vi "校准UI.vi"() -> ()   [LabVIEW 2016, in "斯坦道多参数.lvlib"]
uses:
  <vilib>/Utility/miscctls.llb/LVPointTypeDef.ctl
  <vilib>/Utility/miscctls.llb/LVPositionTypeDef.ctl
  <vilib>/ptbypt/NI_PtbyPt.lvlib
panel:
  out "溶解氧浓度值":dbl=25.0 caption="检测值：" format="%#.2f mg/L"
  out "电极状态标志":u16
  in  "恢复出厂":bool
  in  "电极系数面板":enum32{"选项卡 1"}(tab)
  out "B":dbl=25.0 caption="电极零点：" format="%#.6f"
  out "K":dbl=25.0 caption="电极系数：" format="%#.6f"
  in  "测试参数面板":enum32{"选项卡 1"}(tab)
  in  "自动盐度补偿":bool caption="自动盐度补偿："
  in  "偏移修正值":dbl=25.0 caption="偏移修正值：" format="%#_6f"
  in  "滤波次数":dbl=25.0 caption="滤波次数：" min=1.0 step=1.0
  in  "测量量程":u16(ring)=1 caption="测量量程："
  in  "盐度":dbl=25.0 caption="盐度：" format="%#_6f"
  in  "大气压力":dbl=25.0 caption="大气压力：" format="%#_6f"
  in  "温度系数":dbl=25.0 caption="温度系数：" format="%#.6f"
  out "信号值":dbl=25.0 caption="信号值：" format="%#.2f mV"
  out "检测值":dbl=25.0 caption="检测值：" format="%#.2f"
  out "序列号":string caption="序列号："
  in  "选项卡控件 3":enum32{"选项卡 1"}(tab)
  in  "清扫间隔":u16=25 caption="清扫间隔："
  in  "清扫次数":u16=25 caption="清扫次数："
  in  "清洗":bool caption="探头清洗："
  in  "清扫模式":u16(ring)=1 caption="清扫模式：" items=["自动", "手动"]
  in  "选项卡控件 2":enum32{"选项卡 1"}(tab)
  in  "温度校准系数写入":bool
  in  "温度校准系数读取":bool
  in  "BT":dbl caption="B：" format="%#.6f"
  in  "KT":dbl=1.0 caption="K：" format="%#.6f"
  in  "实际温度":dbl=25.0 caption="校准温度：" format="%.2f ℃"
  out "当前温度":dbl caption="探头温度：" format="%.2f ℃"
  in  "校准温度":bool
  in  "选项卡控件":enum32{"选项卡 1"}(tab)
  in  "第三点确认校准":bool
  in  "第二点确认校准":bool
  in  "标液一":cluster{"标准值":dbl, "检测值":dbl, "原始值":dbl} caption="标液一：" {"原始值" format="%#_6f"; "检测值" format="%#_6f"; "标准值" format="%#.6f"}
  in  "标液二":cluster{"标准值":dbl, "检测值":dbl, "原始值":dbl} caption="标液二：" {"原始值" format="%#_6f"; "检测值" format="%#_6f"; "标准值" format="%#.6f"}
  in  "标液三":cluster{"标准值":dbl, "检测值":dbl, "原始值":dbl} caption="标液三：" {"原始值" format="%#_6f"; "检测值" format="%#_6f"; "标准值" format="%#.6f"}
  in  "标液一开始校准":bool
  in  "第一点确认校准":bool
  in  "标液二开始校准":bool
  in  "标液三开始校准":bool
  in  "显示曲线":bool
  in  "校准记录":string="校准记录\n---------------------------------------------\n序列号：\n温度值：\n标准值：\n检测值：\n原始值：\n校准时间："
  in  "校准方式":u16(ring)=1 caption="校准方式：" items=["单点校准", "两点校准", "三点校准"]
  in  "校准参数":u16(ring) caption="校准参数：" items=["pH", "DO", "浊度", "电导率"]
  # "检测值"
  # "信号值"
  # "标准值"
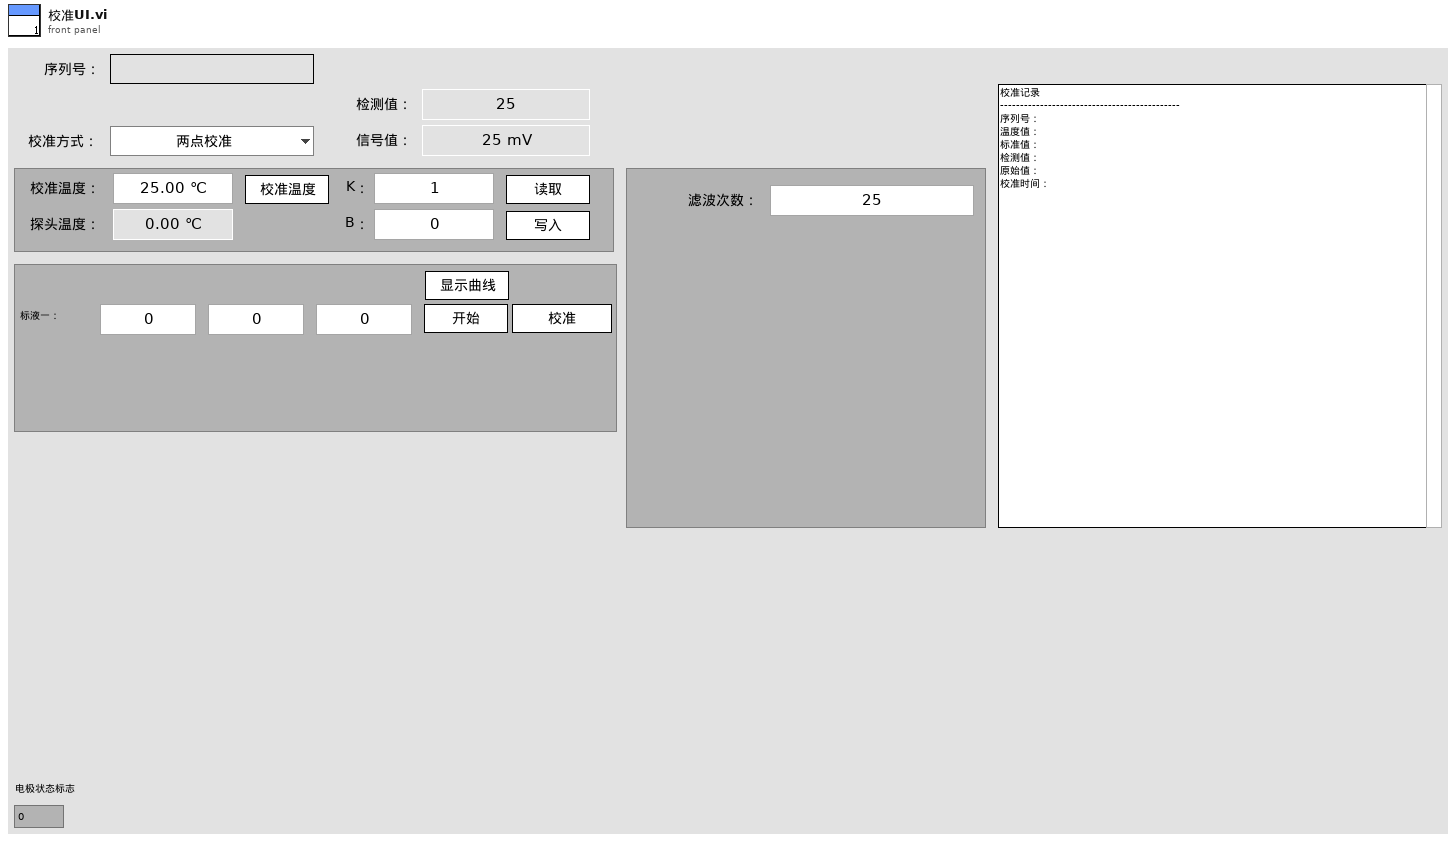
[diagram p1: front panel]
types:
  T1 = typedef "LVPointTypeDef.ctl" = cluster{"Horizontal":i16, "Vertical":i16}
  T2 = cluster{"ph":bool, "DO":bool, "Cond":bool, "Turb":bool, "叶绿素a":bool, "藻密度":bool, "ORP":bool, "COD":bool, "DO2":bool, "氯化物":bool, "氨氮":bool, "水中油":bool, "悬浮物":bool, "余氯":bool}
  T3 = typedef "斯坦道多参数.lvlib/探头类型.ctl" = enum16{"禹山", "国弘", "纳清", "STD"}
  T4 = typedef "LVStringsAndValuesArrayTypeDef_U16.ctl" = cluster{"String":string, "Value":u16}[]
  T5 = enum8{"Enabled", "Disabled", "Disabled and Grayed Out"}
  T6 = typedef "LVPositionTypeDef.ctl" = cluster{"Left":i32, "Top":i32}
  T7 = cluster{"pH":u32, "DO":u32, "Cond":u32, "Turb":u32, "叶绿素a":u32, "藻密度":u32, "ORP":u32, "COD":u32, "氯化物":u32, "氨氮":u32, "水中油":u32, "悬浮物":u32, "余氯":u32}
  T8 = cluster{"电极状态标志":u16, "电极型号标志":u16, "酸碱度测量值":sgl, "温度测量值":sgl, "酸碱度信号值":sgl, "温度信号值":sgl, "酸碱度偏移修正值":sgl, "温度偏移修正值":sgl, "手动温度补偿值":sgl, "酸碱度电极零点":sgl, "酸碱度电极斜率":sgl, "第1点标准值记录":sgl, "第1点信号值记录":sgl, "第1点温度值记录":sgl, "第2点标准值记录":sgl, "第2点信号值记录":sgl, "第2点温度值记录":sgl, "命令滤波设定":u16, "温度模式":enum16{"ATC", "MTC"}, "生产批次":u16, "电极序号":u16, "串口地址":u16, "串口波特率":enum16{"9600", "19200", "115200"}, "串口校验位":enum16{"NONE", "ODD", "EVEN"}, "串口停止位":enum16{"1bit", "2bit"}, "第一点标准值":sgl, "第二点标准值":sgl}
  T9 = cluster{"报警码":u16, "溶解氧数值（mg/L）":sgl, "溶解氧数据（%）":sgl, "温度数据":sgl, "溶解氧原始信号 nA":sgl, "大气压力":sgl, "盐度":sgl, "0X0009_NC":string, "产品名称":string, "序列号":string, "硬件版本":string, "软件版本":string, "通讯地址":u16, "波特率":u16, "设备类型":u16, "0X0026_NC":string, "第一点原始数据":sgl, "第一点校准数据":sgl, "第二点原始数据":sgl, "第二点校准数据":sgl, "探头校准命令":u16, "温度校准参数":sgl, "温度校准命令":u16}
  T10 = cluster{"电极状态标志":u16, "电极型号标志":u16, "溶解氧测量值":sgl, "温度测量值":sgl, "溶解氧饱和度值":sgl, "盐度补偿值":sgl, "大气压补偿值":sgl, "溶解氧偏移修正值":sgl, "温度偏移修正值":sgl, "手动温度补偿值":sgl, "溶解氧电极零点":sgl, "溶解氧电极斜率":sgl, "第1点标准值记录":sgl, "第1点信号值记录":sgl, "第1点温度值记录":sgl, "第2点标准值记录":sgl, "第2点信号值记录":sgl, "第2点温度值记录":sgl, "命令滤波设定":u16, "温度模式":enum16{"ATC", "MTC"}, "生产批次":u16, "电极序号":u16, "串口地址":u16, "串口波特率":enum16{"9600", "19200", "115200"}, "串口校验位":enum16{"NONE", "ODD", "EVEN"}, "串口停止位":enum16{"1bit", "2bit"}, "第一点标准值":sgl, "第二点标准值":sgl}
  T11 = cluster{"电极状态标志":u16, "电极型号标志":u16, "浊度测量值":sgl, "温度测量值":sgl, "浊度信号值":sgl, "浊度偏移修正值":sgl, "温度偏移修正值":sgl, "手动温度补偿值":sgl, "浊度电极零点":sgl, "浊度电极斜率":sgl, "清洁周期":u16, "命令滤波设定":u16, "温度模式":enum16{"ATC", "MTC"}, "生产批次":u16, "电极序号":u16, "串口地址":u16, "串口波特率":enum16{"9600", "19200", "115200"}, "串口校验位":enum16{"NONE", "ODD", "EVEN"}, "串口停止位":enum16{"1bit", "2bit"}, "第一点标准值":sgl, "第二点标准值":sgl, "第三点标准值":sgl}
  T12 = cluster{"报警码":u16, "浊度数值 NTU":sgl, "温度数据":sgl, "原始光强数值":u16, "量程":u16, "平均次数":u16, "清扫模式":u16, "清扫次数":u16, "清扫间隔分钟":u16, "0X000B_NC":string, "产品名称":string, "序列号":string, "硬件版本":string, "软件版本":string, "通讯地址":u16, "波特率":u16, "设备类型":u16, "0X0026_NC":string, "校准量程":u16, "第一点原始光强":u16, "第一点校准数据":sgl, "第二点原始光强":u16, "第二点校准数据":sgl, "第三点原始光强":u16, "第三点校准数据":sgl, "探头校准命令":u16, "温度校准参数":sgl, "温度校准命令":u16}
  T13 = cluster{"电极状态标志":u16, "电极型号标志":u16, "电导率测量值":sgl, "温度测量值":sgl, "电导率信号值":sgl, "温度信号值":sgl, "温度补偿系数":sgl, "电导率偏移修正值":sgl, "温度偏移修正值":sgl, "手动温度补偿值":sgl, "电导率电极零点":sgl, "电导率电极斜率":sgl, "命令滤波设定":u16, "温度模式":enum16{"ATC", "MTC"}, "生产批次":u16, "电极序号":u16, "串口地址":u16, "串口波特率":enum16{"9600", "19200", "115200"}, "串口校验位":enum16{"NONE", "ODD", "EVEN"}, "串口停止位":enum16{"1bit", "2bit"}, "第一点标准值":sgl, "第二点标准值":sgl}
  T14 = cluster{"报警码":u16, "叶绿素a":sgl, "温度数据":sgl, "原始光强数值":u16, "量程":u16, "平均次数":u16, "清扫模式":u16, "清扫次数":u16, "清扫间隔分钟":u16, "0X000B_NC":string, "产品名称":string, "序列号":string, "硬件版本":string, "软件版本":string, "通讯地址":u16, "波特率":u16, "设备类型":u16, "0X0026_NC":string, "校准量程":u16, "第一点原始光强":u16, "第一点校准数据":sgl, "第二点原始光强":u16, "第二点校准数据":sgl, "第三点原始光强":u16, "第三点校准数据":sgl, "探头校准命令":u16, "温度校准参数":sgl, "温度校准命令":u16}
  T15 = cluster{"报警码":u16, "蓝绿藻":sgl, "温度数据":sgl, "原始光强数值":u16, "量程":u16, "平均次数":u16, "清扫模式":u16, "清扫次数":u16, "清扫间隔分钟":u16, "0X000B_NC":string, "产品名称":string, "序列号":string, "硬件版本":string, "软件版本":string, "通讯地址":u16, "波特率":u16, "设备类型":u16, "0X0026_NC":string, "校准量程":u16, "第一点原始光强":u16, "第一点校准数据":sgl, "第二点原始光强":u16, "第二点校准数据":sgl, "第三点原始光强":u16, "第三点校准数据":sgl, "探头校准命令":u16, "温度校准参数":sgl, "温度校准命令":u16}
  T16 = cluster{"电极状态标志":u16, "电极型号标志":u16, "测量值":sgl, "温度测量值":sgl, "信号值":sgl, "温度信号值":sgl, "000AH_NC":sgl, "偏移修正值":sgl, "温度偏移修正值":sgl, "手动温度补偿值":sgl, "命令滤波设定":u16, "温度模式":enum16{"ATC", "MTC"}, "生产批次":u16, "传感器序号":u16, "串口地址":u16, "串口波特率":enum16{"9600", "19200", "115200"}, "串口校验位":enum16{"NONE", "ODD", "EVEN"}, "串口停止位":enum16{"1bit", "2bit"}}
  T17 = cluster{"电极状态标志":u16, "电极型号标志":u16, "COD测量值":sgl, "浊度测量值":sgl, "COD信号值":sgl, "浊度信号值":sgl, "温度测量值":sgl, "COD偏移修正值":sgl, "浊度偏移修正值":sgl, "COD水样校正值":sgl, "温度偏移修正值":sgl, "COD零点系数":sgl, "COD斜率系数":sgl, "浊度零点系数":sgl, "浊度斜率系数":sgl, "COD测值K值":sgl, "浊度测值K值":sgl, "浊度补偿COD系数值":sgl, "COD温度补偿系数值 ":sgl, "测量周期":u16, "清洗周期":u16, "命令寄存器":u16, "数字滤波设定":u16, "温度模式":enum16{"AUTO", "OFF"}, "生产批次":u16, "电极序号":u16, "串口地址":u16, "串口波特率":enum16{"9600", "19200", "115200"}, "串口校验位":enum16{"NONE", "ODD", "EVEN"}, "串口停止位":enum16{"1bit", "2bit"}, "第一点校正指令":u16, "第一点标准值":sgl, "第二点校正指令":u16, "第二点标准值":sgl, "第三点校正指令":u16, "第三点标准值":sgl, "COD吸光度":sgl, "浊度吸光度":sgl, "温度信号值":sgl}
  T18 = cluster{"电极状态标志":u16, "电极型号标志":u16, "测量值":sgl, "温度测量值":sgl, "信号值":sgl, "温度信号值":sgl, "偏移修正值":sgl, "温度偏移修正值":sgl, "手动温度补偿值":sgl, "电极零点":sgl, "电极斜率":sgl, "第1点标准值记录":sgl, "第1点信号值记录":sgl, "第1点温度值记录":sgl, "第2点标准值记录":sgl, "第2点信号值记录":sgl, "第2点温度值记录":sgl, "命令滤波设定":u16, "温度模式":enum16{"ATC", "MTC"}, "生产批次":u16, "电极序号":u16, "串口地址":u16, "串口波特率":enum16{"9600", "19200", "115200"}, "串口校验位":enum16{"NONE", "ODD", "EVEN"}, "串口停止位":enum16{"1bit", "2bit"}, "第一点标准值":sgl, "第二点标准值":sgl}
  T19 = cluster{"电极状态标志":u16, "电极型号标志":u16, "测量值":sgl, "温度测量值":sgl, "信号值":sgl, "水中油B值":sgl, "温度B值":sgl, "水中油零点系数":sgl, "水中油斜率系数":sgl, "水中油K值":sgl, "空白电位值":sgl, "温度信号值":sgl, "温度补偿系数":sgl, "测量档位":u16, "清洁周期":u16, "命令寄存器":u16, "数位滤波设定":u16, "温度模式":enum16{"ATC", "MTC"}, "生产批次":u16, "电极序号":u16, "串口地址":u16, "串口波特率":enum16{"9600", "19200", "115200"}, "串口校验位":enum16{"NONE", "ODD", "EVEN"}, "串口停止位":enum16{"1bit", "2bit"}, "第一点校正指令":u16, "第一点标准值":sgl, "第二点校正指令":u16, "第二点标准值":sgl, "第三点校正指令":u16, "第三点标准值":sgl}
  T20 = enum16{"null", "pH", "DO", "浊度", "电导率", "叶绿素a", "DO2", "藻密度", "悬浮物"}
  T21 = enum16{"null", "pH", "DO", "浊度", "电导率", "叶绿素a", "DO2", "藻密度"}
  T22 = enum16{"null", "pH", "DO", "浊度", "电导率", "叶绿素a", "藻密度"}
  T23 = cluster{"禁用":enum8{"Enabled", "Disabled", "Disabled and Grayed Out"}, "禁用 2":enum8{"Enabled", "Disabled", "Disabled and Grayed Out"}, "禁用 3":enum8{"Enabled", "Disabled", "Disabled and Grayed Out"}}
  T24 = cluster{"ph":bool, "DO":bool, "Cond":bool, "Turb":bool, "叶绿素a":bool, "藻密度":bool, "ORP":bool, "COD":bool, "DO2":bool, bool, "氨氮":bool, "水中油":bool, "悬浮物":bool, "余氯":bool}
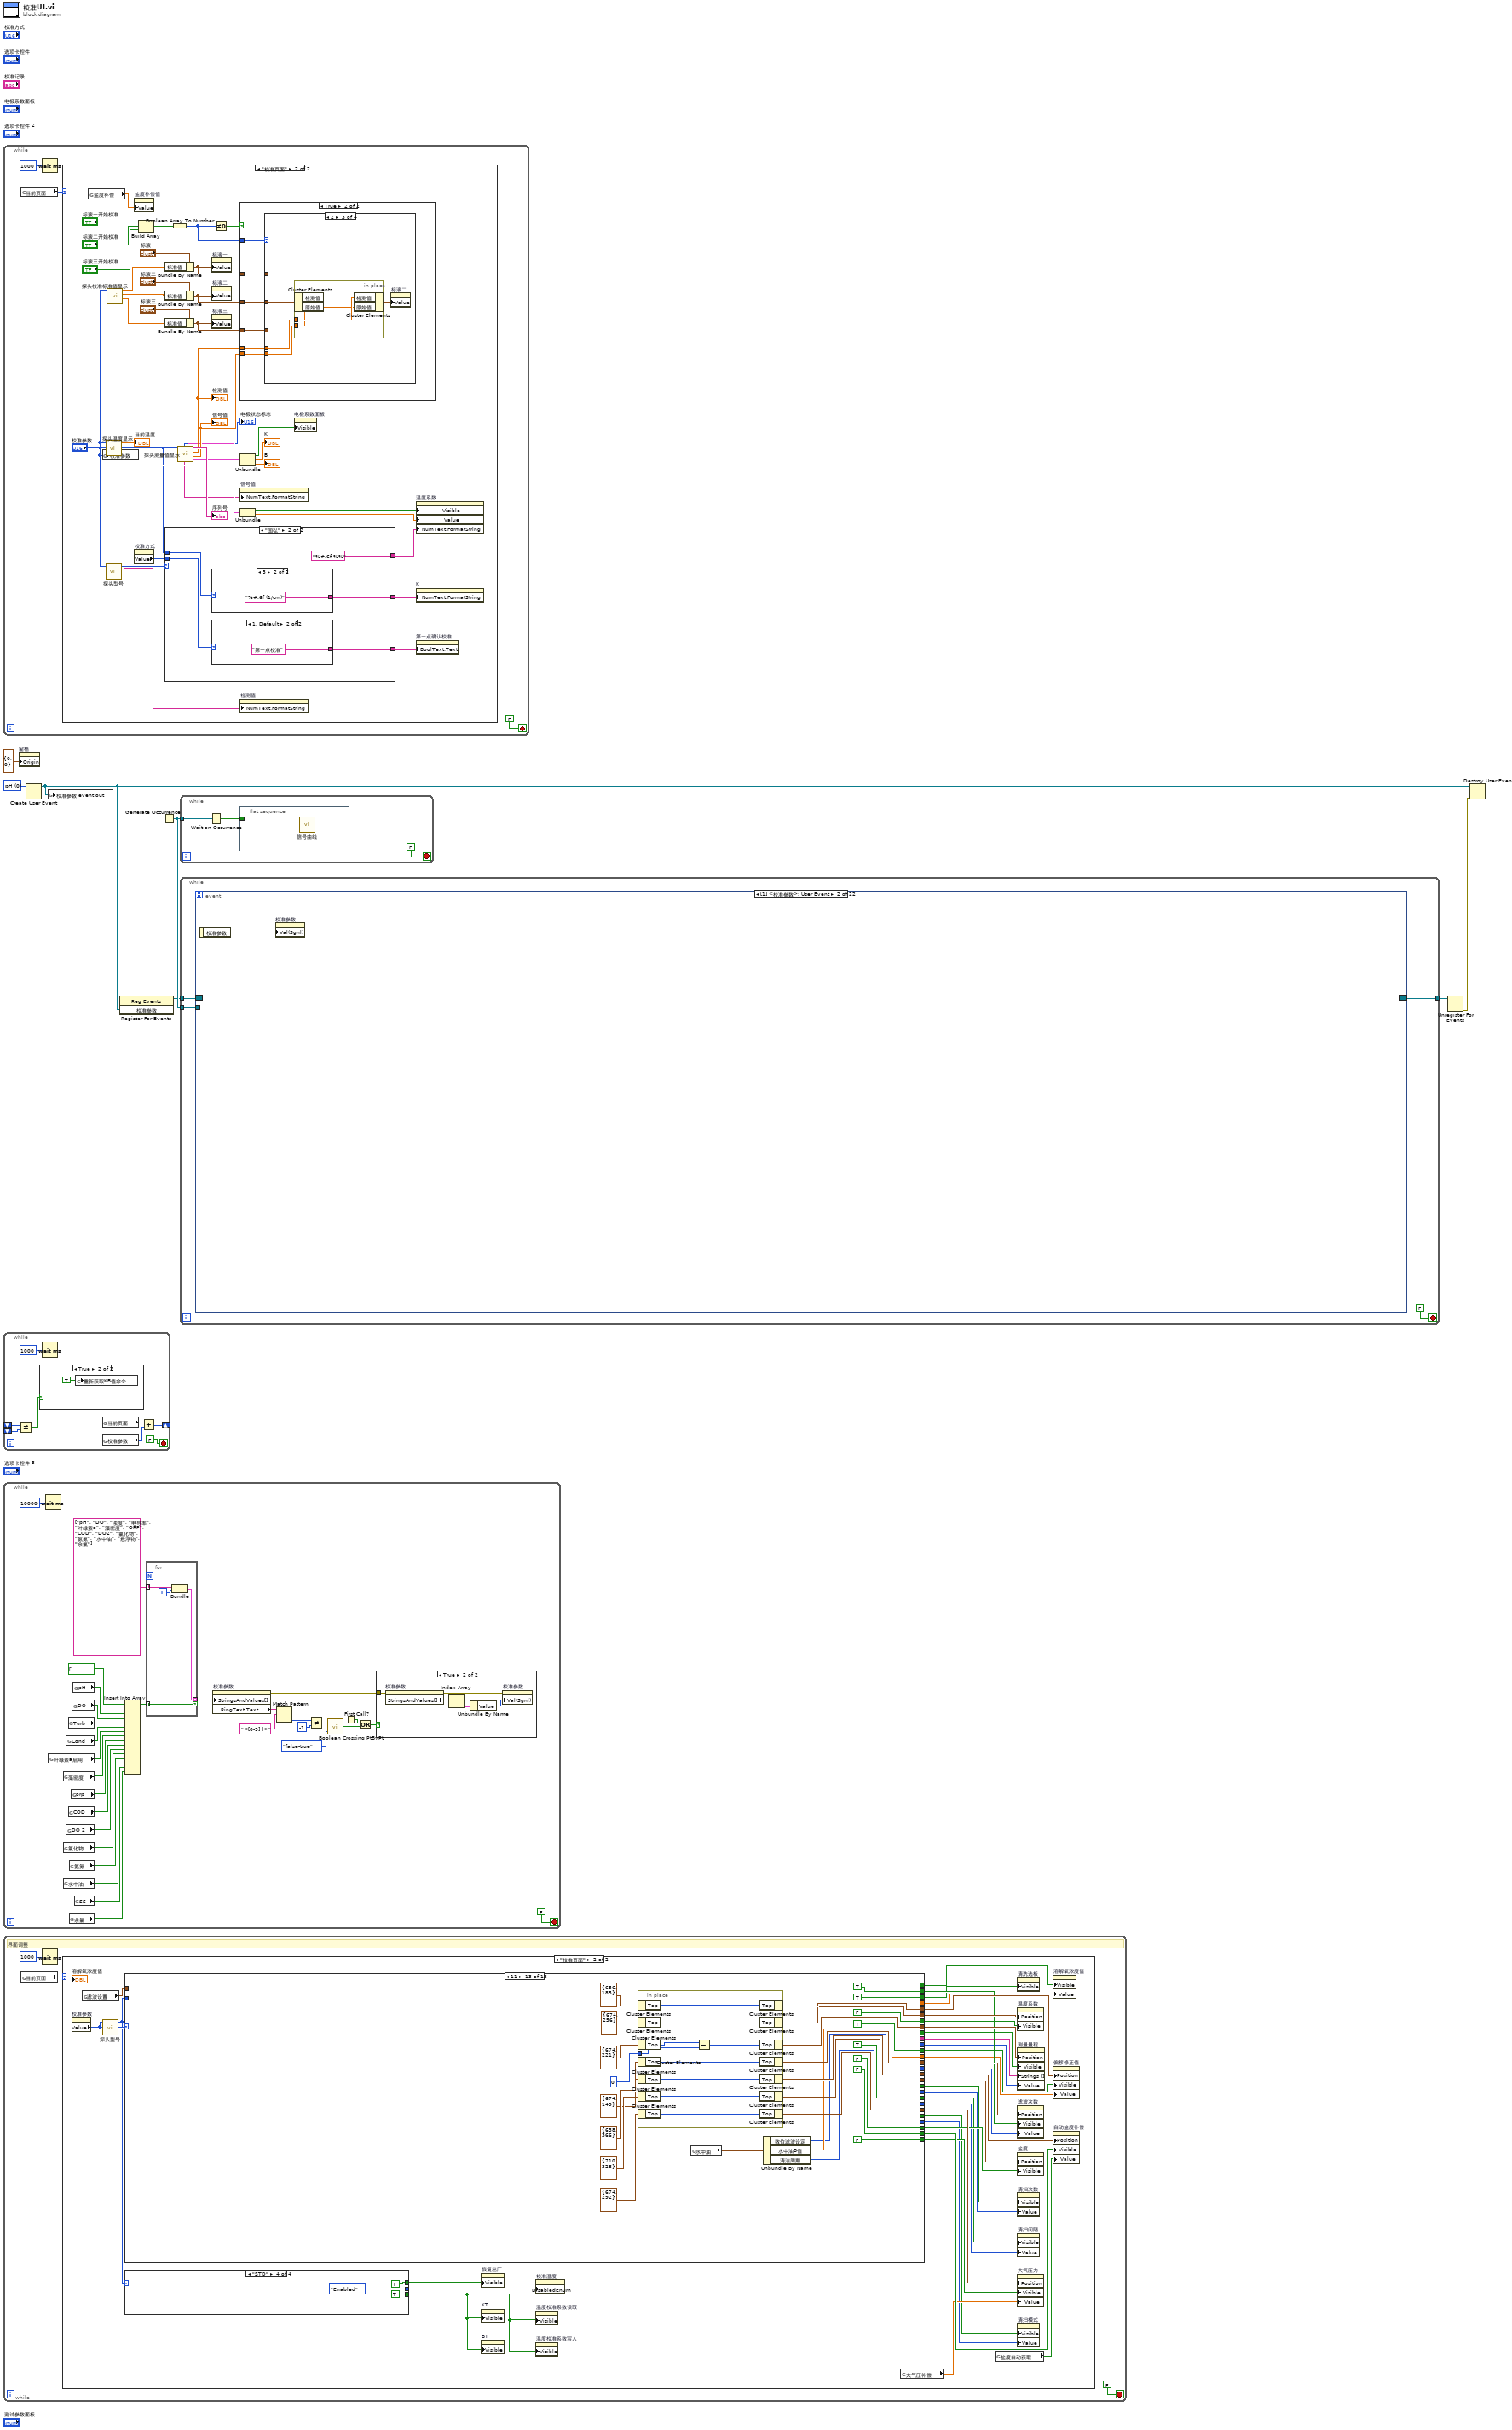
[diagram p0: block diagram]
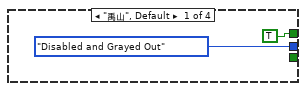
[diagram p4: hidden frame]
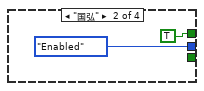
[diagram p5: hidden frame]
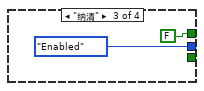
[diagram p6: hidden frame]
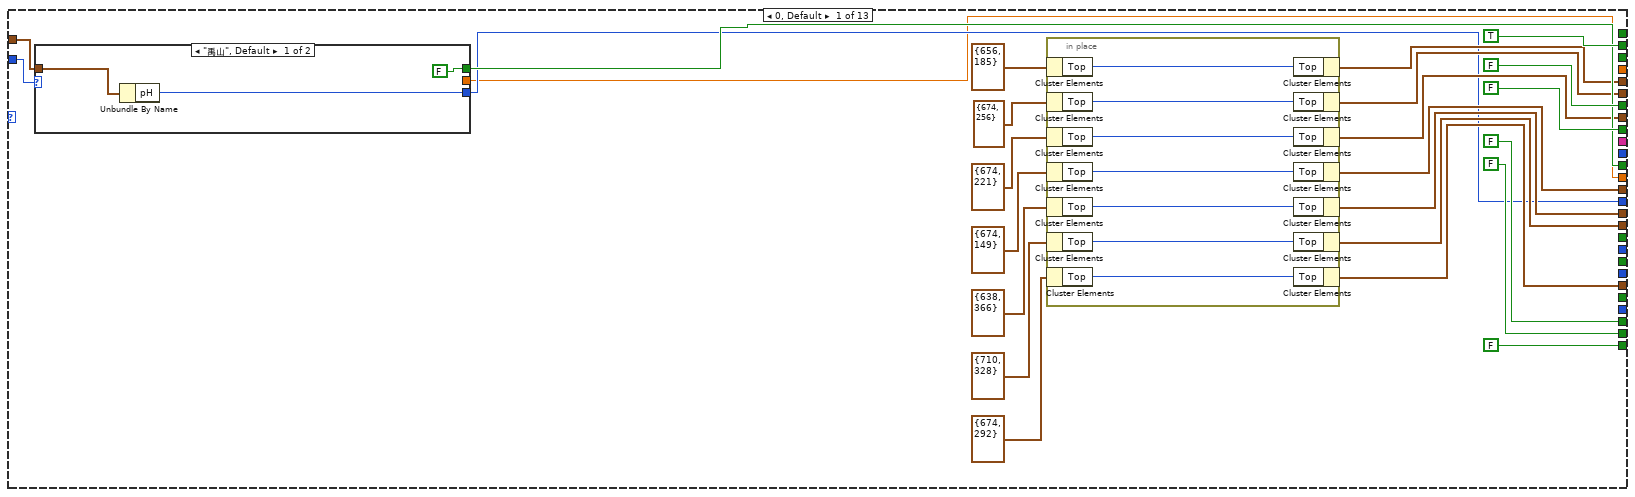
[diagram p7: hidden frame]
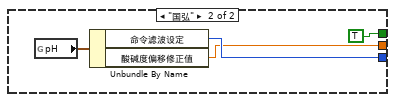
[diagram p8: hidden frame]
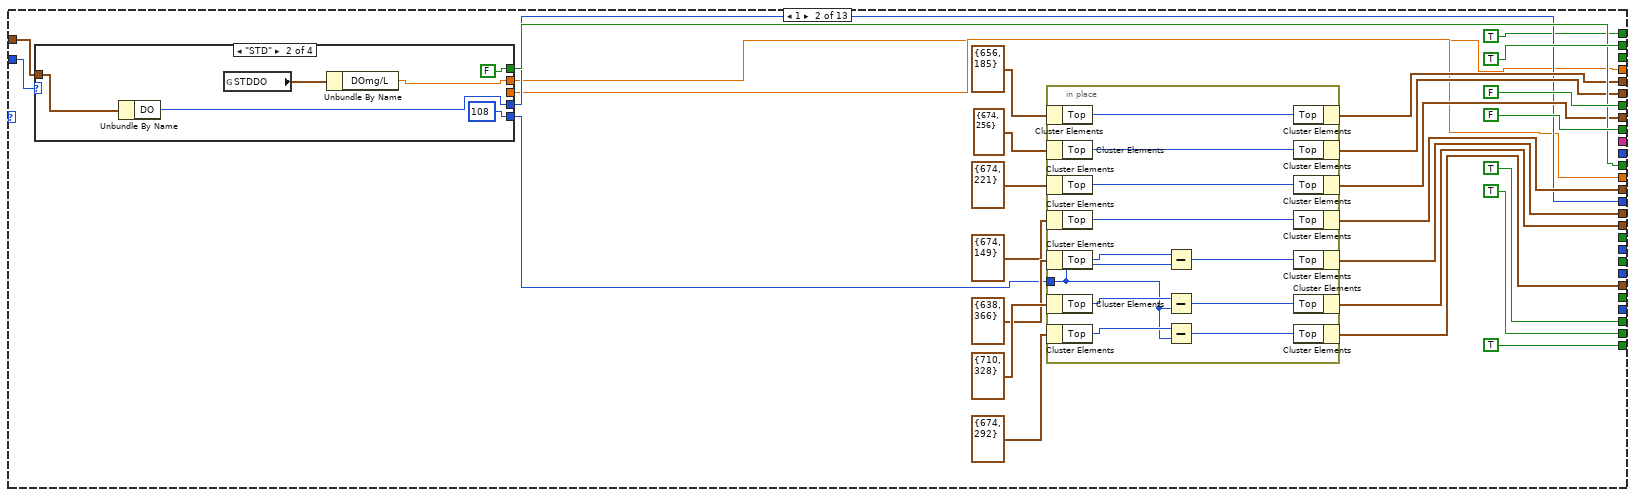
[diagram p9: hidden frame]
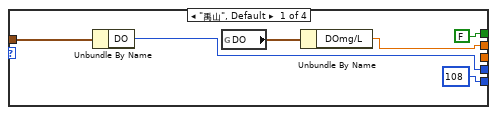
[diagram p10: hidden frame]
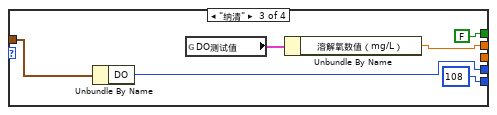
[diagram p11: hidden frame]
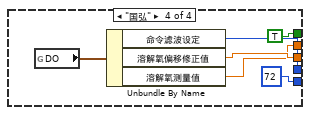
[diagram p12: hidden frame]
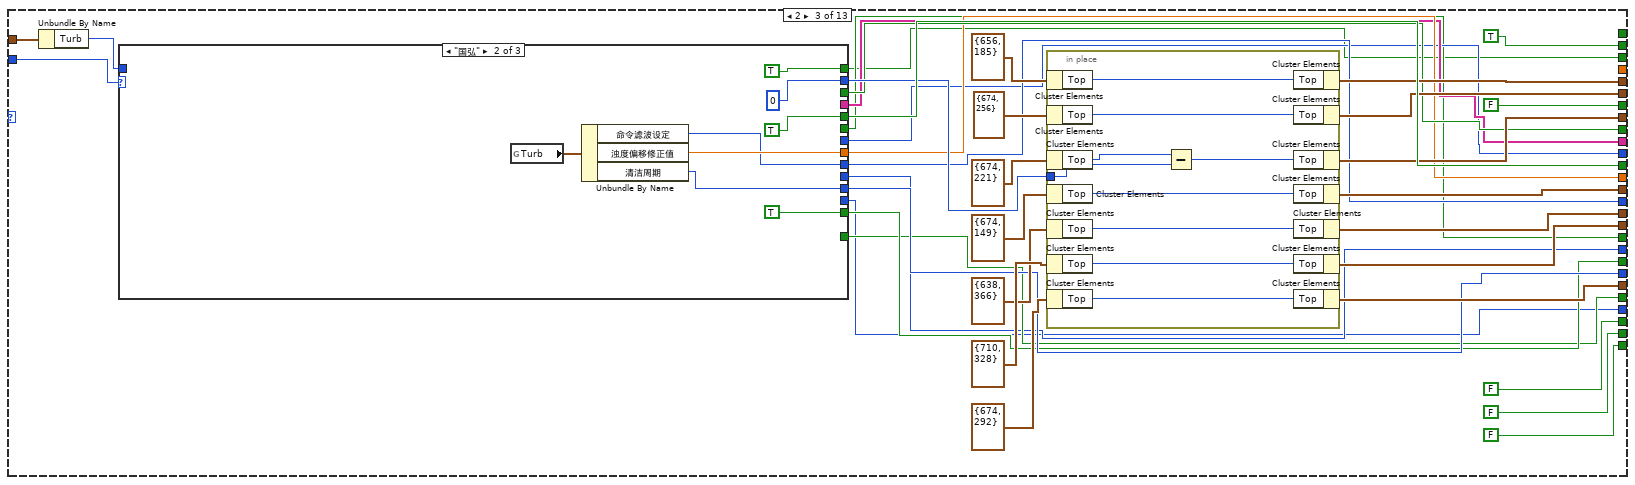
[diagram p13: hidden frame]
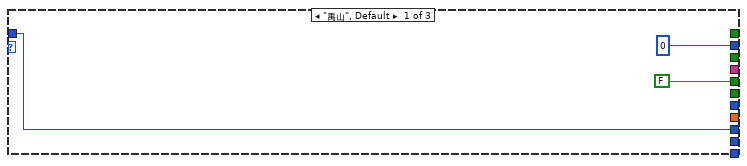
[diagram p14: hidden frame]
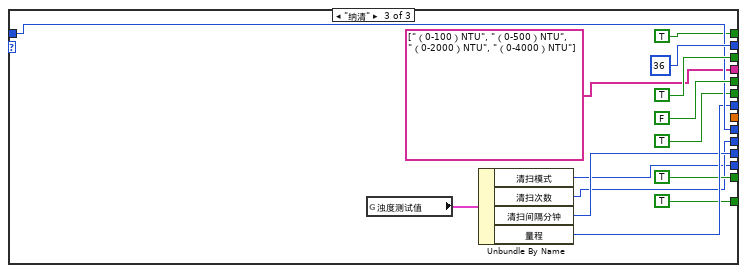
[diagram p15: hidden frame]
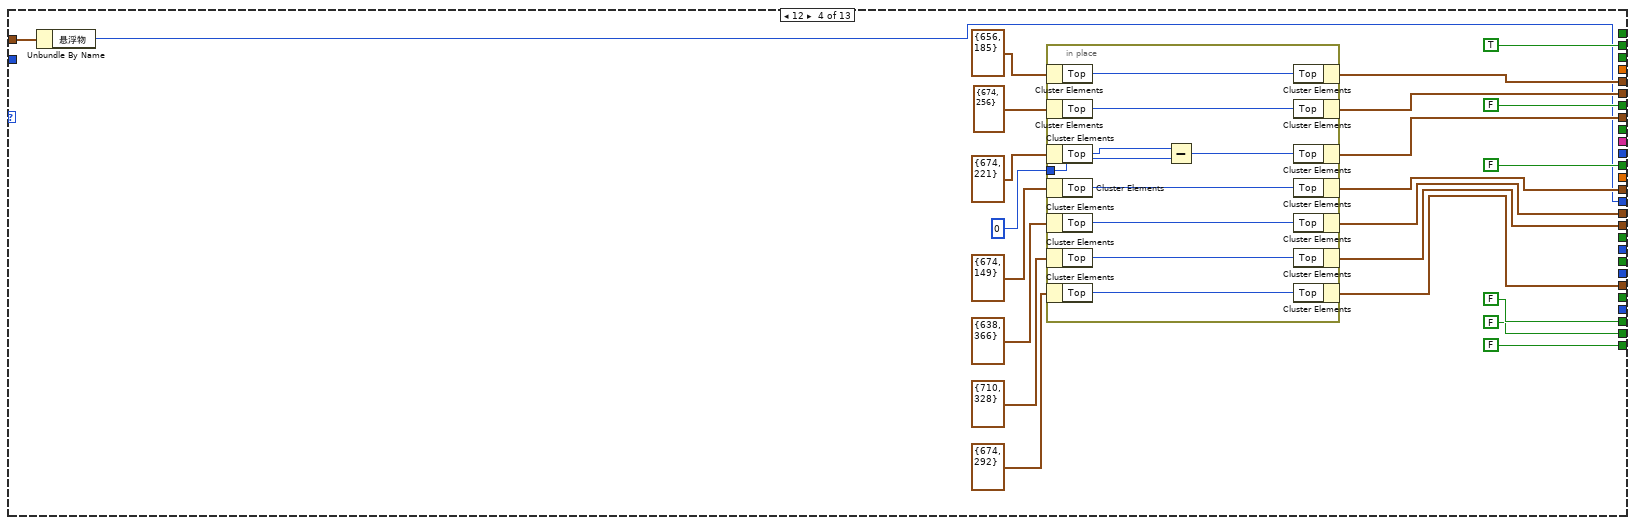
[diagram p16: hidden frame]
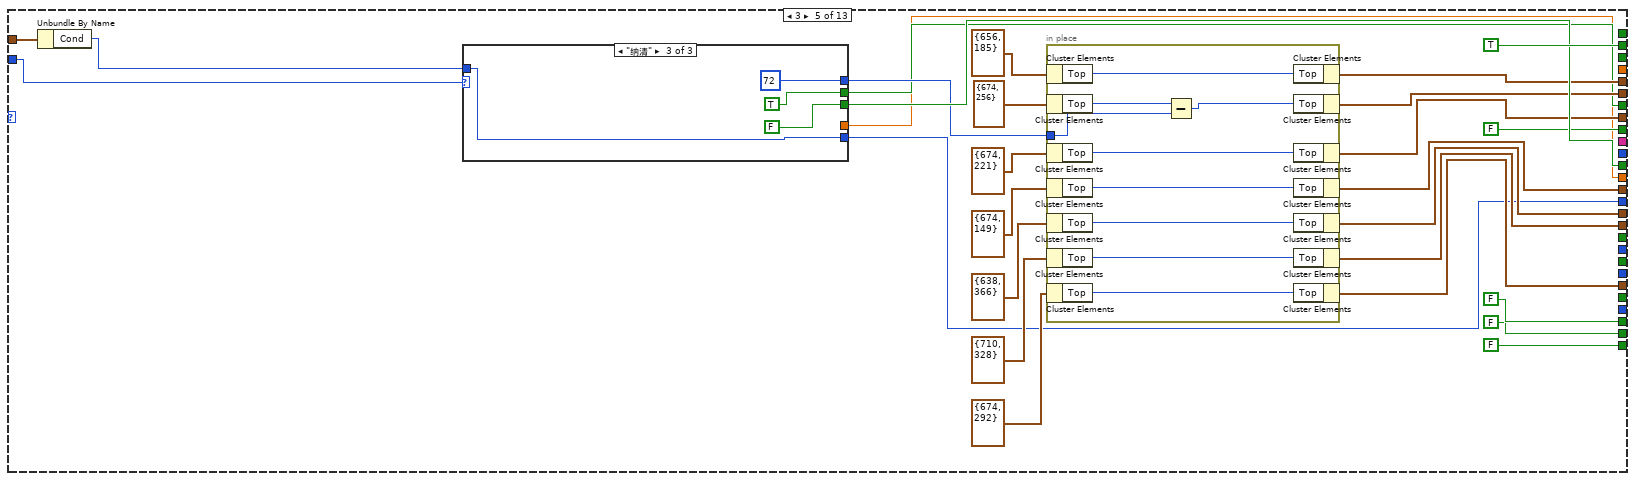
[diagram p17: hidden frame]
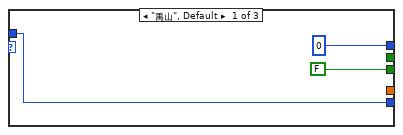
[diagram p18: hidden frame]
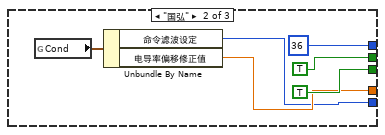
[diagram p19: hidden frame]
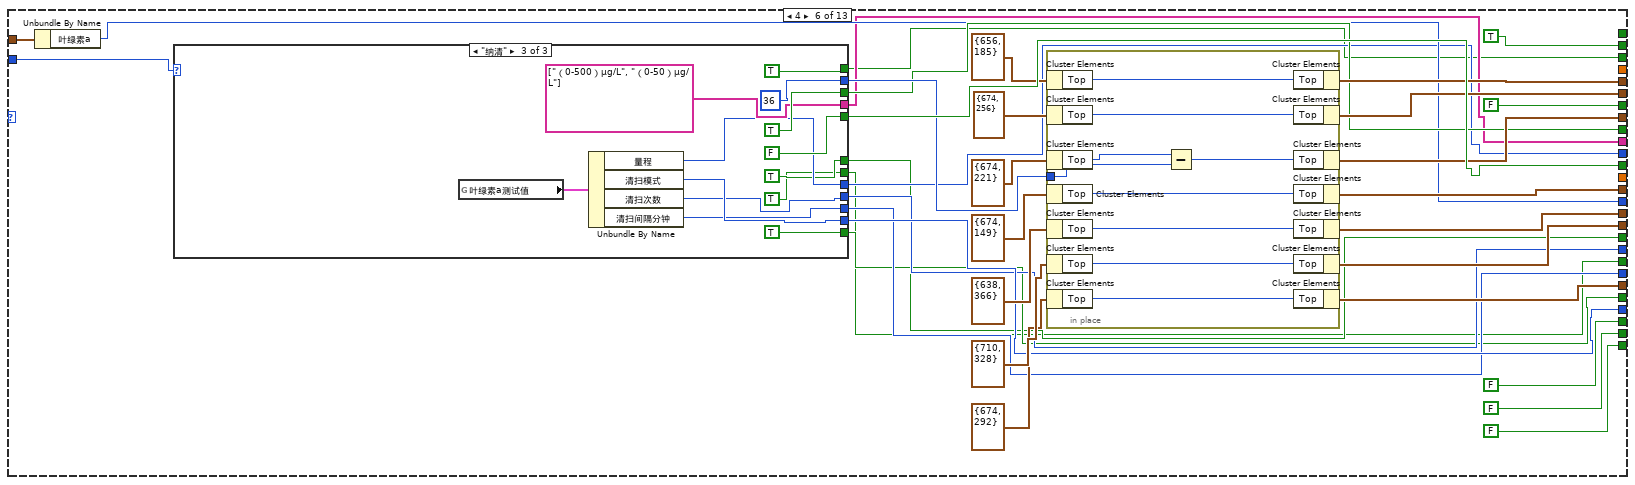
[diagram p20: hidden frame]
diagram:
  w5 = u16 0 items=["pH", "DO", "浊度", "电导率"] ("校准参数")
  n1 = while {
    stop <- FALSE stop-if-true
    n2 = global read "多参数全局变量.vi" "当前页面"() -> (w8:enum16{"主页面", "参数页面", "校准页面"})
    n3 = Wait (ms)(milliseconds to wait=u32 1000 ("等待时间（毫秒）")) -> ()  [unwired: 1 out]
    n4 = case shown="\"校准页面\"" w8 {
      frame "主页面", Default {
        n5 = global write "多参数全局变量.vi" "校准运行状态"(T2 {"ph"=FALSE, "DO"=FALSE, "Cond"=FALSE, "Turb"=FALSE, "叶绿素a"=FALSE, "藻密度"=FALSE, "ORP"=FALSE, "COD"=FALSE, "DO2"=FALSE, "氯化物"=FALSE, "氨氮"=FALSE, "水中油"=FALSE, "悬浮物"=FALSE, "余氯"=FALSE} ("校准运行状态")) -> ()
      }
      frame "校准页面" {
        n6 = global read "断电保存变量.vi" "盐度补偿"() -> (w34:dbl)
        n7 = global write "多参数全局变量.vi" "校准参数"("校准参数") -> ()
        n8 = call "探头温度显示.vi"("校准参数"="校准参数") -> ("温度数据"=→"当前温度":sgl)  [unwired: 9 in, 1 out]
        n9 = call "探头型号.vi"("校准参数"="校准参数") -> ("探头型号"=w29:T3)  [unwired: 8 in, 2 out]
        n10 = call "探头校准标准值显示.vi"("校准参数"="校准参数") -> ("标液三"=w47:sgl, "标液二"=w46:sgl, "标液一"=w45:sgl)  [unwired: 8 in]
        n11 = property on="盐度补偿值" class="DigNum (strict)"("Value"=w34) -> ()  [unwired: 2 in, 2 out]
        n12 = property on="校准方式" class="Ring (strict)"() -> ("Value"=w27:u16)  [unwired: 2 in, 2 out]
        n13 = Build Array("标液一开始校准", "标液二开始校准", "标液三开始校准") -> (w15:bool[])
        n14 = Bundle By Name(cluster="标液一", "标准值"=w45) -> (w41:cluster{"标准值":dbl, "检测值":dbl, "原始值":dbl})
        n15 = Bundle By Name(cluster="标液二", "标准值"=w46) -> (w40:cluster{"标准值":dbl, "检测值":dbl, "原始值":dbl})
        n16 = Bundle By Name(cluster="标液三", "标准值"=w47) -> (w39:cluster{"标准值":dbl, "检测值":dbl, "原始值":dbl})
        n17 = case shown="\"国弘\"" w29 {
          tunnel: ["校准" w55] -> w28
          tunnel: w27 -> [_ w54]
          tunnel: "校准参数" -> [_ w53]
          tunnel: ["%#.6f" ("数值文本.格式字符串") w52] -> w20
          tunnel: ["%#.6f" ("数值文本.格式字符串") "%#.6f %%" ("数值文本.格式字符串")] -> w19
          frame "禹山", Default {
          }
          frame "国弘" {
            n18 = case shown="3" w53 {
              tunnel: ["%#.6f" ("数值文本.格式字符串") "%#.6f (1/cm)" ("数值文本.格式字符串")] -> w52
              frame 0, Default {
              }
              frame 3 {
              }
            }
            n19 = case shown="1, Default" w54 {
              tunnel: ["校准" "第一点校准"] -> w55
              frame 0 {
              }
              frame 1, Default {
              }
            }
          }
        }
        n20 = Boolean Array To Number(Boolean array=w15) -> (number=w13:u32)
        n21 = call "探头测量值显示.vi"("校准参数"="校准参数") -> ("线性系数"=w33:cluster{bool, "K":sgl, "B":sgl}, "信号值"=w35:sgl, "检测值"=w36:sgl, "序列号"=→"序列号":string, "检测值.格式字符串"=w26:string, "温度补偿系数"=w25:cluster{bool, "温度补偿系数":sgl}, "信号值.格式字符串"=w21:string, "电极状态标志"=→"电极状态标志":u16)  [unwired: 3 in]
        "检测值" <- w36
        "信号值" <- w35
        n22 = property on="标液一" class="Clust (strict)"("Value"=w41) -> ()  [unwired: 2 in, 2 out]
        n23 = property on="标液二" class="Clust (strict)"("Value"=w40) -> ()  [unwired: 2 in, 2 out]
        n24 = property on="标液三" class="Clust (strict)"("Value"=w39) -> ()  [unwired: 2 in, 2 out]
        n25 = Not Equal To 0?(x=w13) -> (x != 0?=w14:bool)
        n26 = case shown="True" w14 {
          tunnel: w41 -> [_ w65]
          tunnel: w40 -> [_ w64]
          tunnel: w39 -> [_ w63]
          tunnel: w35 -> [_ w62]
          tunnel: w36 -> [_ w61]
          tunnel: w13 -> [_ w60]
          frame False {
          }
          frame True {
            n27 = case shown="2" w60 {
              tunnel: w61 -> [_ w68 w75 w81]
              tunnel: w62 -> [_ w67 w74 w80]
              tunnel: w65 -> [_ w69 _ _]
              tunnel: w64 -> [_ _ w72 _]
              tunnel: w63 -> [_ _ _ w78]
              frame Default {
              }
              frame 1 {
                n28 = in-place {
                  in-place-border: w68 -> [w71]
                  in-place-border: w67 -> [w70]
                  n29 = in-place-cluster #1(w69) -> ()  [unwired: 2 out]
                  n30 = in-place-cluster #1("检测值"=w71, "原始值"=w70) -> (w66:cluster{"标准值":dbl, "检测值":dbl, "原始值":dbl})
                }
                n31 = property on="标液一" class="Clust (strict)"("Value"=w66) -> ()  [unwired: 2 in, 2 out]
              }
              frame 2 {
                n32 = in-place {
                  in-place-border: w75 -> [w77]
                  in-place-border: w74 -> [w76]
                  n33 = in-place-cluster #2(w72) -> ()  [unwired: 2 out]
                  n34 = in-place-cluster #2("检测值"=w77, "原始值"=w76) -> (w73:cluster{"标准值":dbl, "检测值":dbl, "原始值":dbl})
                }
                n35 = property on="标液二" class="Clust (strict)"("Value"=w73) -> ()  [unwired: 2 in, 2 out]
              }
              frame 4 {
                n36 = in-place {
                  in-place-border: w81 -> [w83]
                  in-place-border: w80 -> [w82]
                  n37 = in-place-cluster #3(w78) -> ()  [unwired: 2 out]
                  n38 = in-place-cluster #3("检测值"=w83, "原始值"=w82) -> (w79:cluster{"标准值":dbl, "检测值":dbl, "原始值":dbl})
                }
                n39 = property on="标液三" class="Clust (strict)"("Value"=w79) -> ()  [unwired: 2 in, 2 out]
              }
            }
          }
        }
        n40 = Unbundle(w33) -> (w32:bool, "K"=→"K":sgl, "B"=→"B":sgl)
        n41 = property on="信号值" class="DigNum (strict)"("NumText.FormatString"=w21) -> ()  [unwired: 2 in, 2 out]
        n42 = Unbundle(w25) -> (w24:bool, "温度补偿系数"=w23:sgl)
        n43 = property on="检测值" class="DigNum (strict)"("NumText.FormatString"=w26) -> ()  [unwired: 2 in, 2 out]
        n44 = property on="电极系数面板" class="TabCtl (strict)"("Visible"=w32) -> ()  [unwired: 2 in, 2 out]
        n45 = property on="温度系数" class="DigNum (strict)"("Visible"=w24, "Value"=w23, "NumText.FormatString"=w19) -> ()  [unwired: 2 in, 2 out]
        n46 = property on="K" class="DigNum (strict)"("NumText.FormatString"=w20) -> ()  [unwired: 2 in, 2 out]
        n47 = property on="第一点确认校准" class="Bool"("BoolText.Text"=w28) -> ()  [unwired: 2 in, 2 out]
      }
    }
  }
  n48 = while {
    shift-right: [w87] -> _
    shift-left: _ -> [w86]
    shift-left: _ -> [w85]
    stop <- FALSE stop-if-true
    n49 = Not Equal?(x=w86, y=w85) -> (x != y?=w84:bool)
    n50 = case shown="True" w84 {
      frame False {
      }
      frame True {
        n51 = global write "多参数全局变量.vi" "重新获取KB值命令"(TRUE ("重新获取KB值命令")) -> ()
      }
    }
    n52 = Wait (ms)(milliseconds to wait=u32 1000 ("等待时间（毫秒）")) -> ()  [unwired: 1 out]
    n53 = global read "多参数全局变量.vi" "当前页面"() -> (w88:enum16{"主页面", "参数页面", "校准页面"})
    n54 = global read "多参数全局变量.vi" "校准参数"() -> (w89:u16)
    n55 = Add(x=w88, y=w89) -> (x+y=w87:u16)
  }
  n56 = while {
    stop <- FALSE stop-if-true
    n57 = Wait (ms)(milliseconds to wait=u32 10000 ("等待时间（毫秒）")) -> ()  [unwired: 1 out]
    n58 = global read "断电保存变量.vi" "叶绿素a启用"() -> (w102:bool)
    n59 = global read "断电保存变量.vi" "藻密度"() -> (w101:bool)
    n60 = global read "断电保存变量.vi" "氯化物"() -> (w97:bool)
    n61 = global read "断电保存变量.vi" "水中油"() -> (w95:bool)
    n62 = global read "断电保存变量.vi" "Cond"() -> (w103:bool)
    n63 = global read "断电保存变量.vi" "DO 2"() -> (w98:bool)
    n64 = global read "断电保存变量.vi" "Turb"() -> (w119:bool)
    n65 = global read "断电保存变量.vi" "COD"() -> (w99:bool)
    n66 = global read "断电保存变量.vi" "氨氮"() -> (w96:bool)
    n67 = global read "断电保存变量.vi" "余氯"() -> (w93:bool)
    n68 = global read "断电保存变量.vi" "orp"() -> (w100:bool)
    n69 = global read "断电保存变量.vi" "DO"() -> (w120:bool)
    n70 = global read "断电保存变量.vi" "pH"() -> (w122:bool)
    n71 = global read "断电保存变量.vi" "SS"() -> (w94:bool)
    n72 = Insert Into Array(array=bool[] [] ("数组"), new element #1=w122, new element #2=w120, new element #3=w119, new element #4=w103, new element #5=w102, new element #6=w101, new element #7=w100, new element #8=w99, new element #9=w98, new element #10=w97, new element #11=w96, new element #12=w95, new element #13=w94, new element #14=w93) -> (w116:bool[])  [unwired: 1 in]
    n73 = for {
      tunnel: w116 -> [w128] mode=indexing
      tunnel: string[] ["pH", "DO", "浊度", "电导率", "叶绿素a", "藻密度", "ORP", "COD", "DO2", "氯化物", "氨氮", "水中油", "悬浮物", "余氯"] ("字符串[]") -> [w130] mode=indexing
      tunnel: [w129] -> w113 mode=indexing if=w128
      i -> [w131]
      n74 = Bundle(w130, w131) -> (w129:cluster{string, i32})  [unwired: 1 in]
    }
    n75 = property on="校准参数" class="Ring (strict)"("StringsAndValues[]"=w113) -> (error out=w114:errorcluster, "RingText.Text"=w112:string)  [unwired: 2 in, 1 out]
    n76 = Match Pattern(string=w112, regular expression="<[0-9]+>" ("正则表达式")) -> (offset past match=w110:i32)  [unwired: 1 in, 3 out]
    n77 = Not Equal?(x=w110, y=-1) -> (x != y?=w108:bool)
    n78 = call <vilib>:"Boolean Crossing PtByPt.vi"("direction"=enum16{"either", "false-true", "true-false"}."false-true", "input"=w108) -> ("crossing"=w105:bool)  [unwired: 1 in]
    n79 = First Call?() -> (First Call?: T/F=w106:bool)
    n80 = Or(x=w106, y=w105) -> (x .or. y?=w107:bool)
    n81 = case shown="True" w107 {
      tunnel: w114 -> [_ w127]
      frame False {
      }
      frame True {
        n82 = property on="校准参数" class="Ring (strict)"(error in=w127) -> (error out=w126:errorcluster, "StringsAndValues[]"=w125:T4)  [unwired: 1 in, 1 out]
        n83 = Index Array(array=w125) -> (element=w124:cluster{"String":string, "Value":u16})  [unwired: 1 in]
        n84 = Unbundle By Name(w124) -> ("Value"=w123:u16)
        n85 = property on="校准参数" class="Ring (strict)"(error in=w126, "Val(Sgnl)"=w123) -> ()  [unwired: 1 in, 2 out]
      }
    }
  }
  n86 = while {
    stop <- FALSE stop-if-true
    # "界面调整"
    n87 = global read "多参数全局变量.vi" "当前页面"() -> (w133:enum16{"主页面", "参数页面", "校准页面"})
    n88 = Wait (ms)(milliseconds to wait=u32 1000 ("等待时间（毫秒）")) -> ()  [unwired: 1 out]
    n89 = case shown="\"校准页面\"" w133 {
      frame "主页面", Default {
      }
      frame "校准页面" {
        n90 = property on="校准参数" class="Ring (strict)"() -> ("Value"=w168:u16)  [unwired: 2 in, 2 out]
        n91 = global read "断电保存变量.vi" "滤波设置"() -> (w150:T7)
        n92 = call "探头型号.vi"("校准参数"=w168) -> ("探头型号"=w138:T3)  [unwired: 8 in, 2 out]
        n93 = case shown="11" w168 {
          tunnel: [w188 w229 w301 w359 w395 w450 w510 w562 w600 w633 w674 w704 w738] -> w169
          tunnel: w138 -> [w196 w238 w310 _ w404 w459 w519 w570 _ w642 _ _ _]
          tunnel: [w186 w227 w299 w357 w393 w448 w508 w560 w598 w631 w672 w702 w736] -> w167
          tunnel: [w184 w225 w297 w355 w391 w446 w506 w558 w596 w629 w670 w700 w734] -> w166
          tunnel: [w182 w223 w295 w353 w389 w444 w504 w556 w594 w627 w668 w698 w732] -> w165
          tunnel: [w190 w231 w303 w361 w397 w452 w512 w564 w602 w635 w676 w706 w740] -> w164
          tunnel: [w192 w234 w306 w364 w400 w455 w515 w566 w604 w638 w678 w708 w743] -> w163
          tunnel: [w191 w232 w304 w362 w398 w453 w513 w565 w603 w636 w677 w707 w741] -> w162
          tunnel: [TRUE TRUE TRUE TRUE TRUE TRUE TRUE TRUE TRUE TRUE TRUE TRUE TRUE] -> w161
          tunnel: [FALSE FALSE w294 _ FALSE w443 w503 FALSE FALSE FALSE FALSE FALSE _] -> w160
          tunnel: [FALSE TRUE FALSE FALSE FALSE FALSE FALSE FALSE FALSE TRUE FALSE FALSE FALSE] -> w159
          tunnel: [FALSE FALSE FALSE FALSE w387 FALSE FALSE FALSE FALSE FALSE FALSE FALSE FALSE] -> w158
          tunnel: [w199 w241 w313 FALSE w407 w462 w522 w573 TRUE w645 TRUE FALSE TRUE] -> w157
          tunnel: [FALSE TRUE FALSE FALSE FALSE FALSE FALSE FALSE FALSE TRUE FALSE FALSE FALSE] -> w156
          tunnel: [FALSE TRUE FALSE FALSE FALSE FALSE FALSE FALSE FALSE TRUE FALSE FALSE FALSE] -> w155
          tunnel: [w181 w221 w292 w351 w384 w441 w501 w554 w593 w625 w667 w697 w730] -> w152
          tunnel: [w180 w220 w293 _ w383 _ _ w555 w592 _ w666 _ w731] -> w151
          tunnel: w150 -> [w179 w222 w291 w352 w386 w442 w502 w553 _ w626 _ w696 _]
          tunnel: [_ _ w289 _ _ w440 w500 _ _ _ _ _ _] -> w149
          tunnel: [_ _ w288 _ _ w439 w499 _ _ _ _ _ _] -> w148
          tunnel: [_ _ w287 _ _ w436 w495 _ _ _ _ _ w729] -> w147
          tunnel: [_ _ w286 _ _ w433 w493 _ _ _ _ _ TRUE] -> w146
          tunnel: [_ _ w285 _ _ w434 w492 _ _ _ _ _ _] -> w145
          tunnel: [_ _ w284 _ _ w435 w494 _ _ _ _ _ _] -> w144
          tunnel: [_ _ w283 _ _ w437 w496 _ _ _ _ _ _] -> w143
          tunnel: [_ _ w282 _ _ w438 w497 _ _ _ _ _ _] -> w142
          tunnel: [_ _ w281 _ _ w432 w498 _ _ _ _ _ TRUE] -> w141
          tunnel: [_ w219 _ _ _ _ _ _ _ w623 _ _ _] -> w139
          tunnel: [_ TRUE _ _ _ _ _ _ _ TRUE _ _ _] -> w140
          frame 0, Default {
            n94 = case shown="\"禹山\", Default" w196 {
              tunnel: [FALSE TRUE] -> w199
              tunnel: [w211 w215] -> w181
              tunnel: [_ w214] -> w180
              tunnel: w179 -> [w212 _]
              frame "禹山", Default {
                n95 = Unbundle By Name(w212) -> ("pH"=w211:u32)
              }
              frame "国弘" {
                n96 = global read "国弘过程全局变量.vi" "pH"() -> (w216:T8)
                n97 = Unbundle By Name(w216) -> ("命令滤波设定"=w215:u16, "酸碱度偏移修正值"=w214:sgl)
              }
            }
            n98 = in-place {
              n99 = in-place-cluster #4(T6 {"Left"=656, "Top"=185} ("位置 2")) -> ("Top"=w209:i32)
              n100 = in-place-cluster #5(T6 {"Left"=674, "Top"=256} ("位置 4")) -> ("Top"=w208:i32)
              n101 = in-place-cluster #6(T6 {"Left"=674, "Top"=221} ("位置 3")) -> ("Top"=w207:i32)
              n102 = in-place-cluster #7(T6 {"Left"=674, "Top"=149} ("位置")) -> ("Top"=w210:i32)
              n103 = in-place-cluster #8(T6 {"Left"=638, "Top"=366} ("位置 7")) -> ("Top"=w204:i32)
              n104 = in-place-cluster #9(T6 {"Left"=710, "Top"=328} ("位置 6")) -> ("Top"=w205:i32)
              n105 = in-place-cluster #10(T6 {"Left"=674, "Top"=292} ("位置 5")) -> ("Top"=w206:i32)
              n106 = in-place-cluster #4("Top"=w209) -> (w186:T6)
              n107 = in-place-cluster #5("Top"=w208) -> (w182:T6)
              n108 = in-place-cluster #6("Top"=w207) -> (w184:T6)
              n109 = in-place-cluster #7("Top"=w210) -> (w188:T6)
              n110 = in-place-cluster #8("Top"=w204) -> (w191:T6)
              n111 = in-place-cluster #9("Top"=w205) -> (w192:T6)
              n112 = in-place-cluster #10("Top"=w206) -> (w190:T6)
            }
          }
          frame 1 {
            n113 = case shown="\"STD\"" w238 {
              tunnel: [FALSE FALSE FALSE TRUE] -> w241
              tunnel: [108 ("y") 108 ("y") 108 ("y") 72 ("y")] -> w233
              tunnel: w222 -> [w260 w266 w272 _]
              tunnel: [w259 w265 w271 w276] -> w221
              tunnel: [_ _ _ w277] -> w220
              tunnel: [w257 w263 w269 w275] -> w219
              frame "禹山", Default {
                n114 = Unbundle By Name(w260) -> ("DO"=w259:u32)
                n115 = global read "禹山过程全局变量.vi" "DO"() -> (w258:cluster{"温度测量值":sgl, "DO%":sgl, "DOmg/L":sgl})
                n116 = Unbundle By Name(w258) -> ("DOmg/L"=w257:sgl)
              }
              frame "STD" {
                n117 = Unbundle By Name(w266) -> ("DO"=w265:u32)
                n118 = global read "禹山过程全局变量.vi" "STDDO"() -> (w264:cluster{"温度测量值":sgl, "DO%":sgl, "DOmg/L":sgl})
                n119 = Unbundle By Name(w264) -> ("DOmg/L"=w263:sgl)
              }
              frame "纳清" {
                n120 = Unbundle By Name(w272) -> ("DO"=w271:u32)
                n121 = global read "纳清过程全局变量.vi" "DO测试值"() -> (w270:T9)
                n122 = Unbundle By Name(w270) -> ("溶解氧数值（mg/L）"=w269:sgl)
              }
              frame "国弘" {
                n123 = global read "国弘过程全局变量.vi" "DO"() -> (w278:T10)
                n124 = Unbundle By Name(w278) -> ("命令滤波设定"=w276:u16, "溶解氧偏移修正值"=w277:sgl, "溶解氧测量值"=w275:sgl)
              }
            }
            n125 = in-place {
              in-place-border: w233 -> [w250]
              n126 = in-place-cluster #11(T6 {"Left"=656, "Top"=185} ("位置 2")) -> ("Top"=w248:i32)
              n127 = in-place-cluster #12(T6 {"Left"=674, "Top"=256} ("位置 4")) -> ("Top"=w247:i32)
              n128 = in-place-cluster #13(T6 {"Left"=674, "Top"=221} ("位置 3")) -> ("Top"=w246:i32)
              n129 = in-place-cluster #14(T6 {"Left"=674, "Top"=149} ("位置")) -> ("Top"=w249:i32)
              n130 = in-place-cluster #15(T6 {"Left"=638, "Top"=366} ("位置 7")) -> ("Top"=w254:i32)
              n131 = in-place-cluster #16(T6 {"Left"=710, "Top"=328} ("位置 6")) -> ("Top"=w256:i32)
              n132 = in-place-cluster #17(T6 {"Left"=674, "Top"=292} ("位置 5")) -> ("Top"=w252:i32)
              n133 = Subtract(x=w254, y=w250) -> (x-y=w253:i32)
              n134 = Subtract(x=w256, y=w250) -> (x-y=w255:i32)
              n135 = Subtract(x=w252, y=w250) -> (x-y=w251:i32)
              n136 = in-place-cluster #11("Top"=w248) -> (w227:T6)
              n137 = in-place-cluster #12("Top"=w247) -> (w223:T6)
              n138 = in-place-cluster #13("Top"=w246) -> (w225:T6)
              n139 = in-place-cluster #14("Top"=w249) -> (w229:T6)
              n140 = in-place-cluster #15("Top"=w253) -> (w232:T6)
              n141 = in-place-cluster #16("Top"=w255) -> (w234:T6)
              n142 = in-place-cluster #17("Top"=w251) -> (w231:T6)
            }
          }
          frame 2 {
            n143 = Unbundle By Name(w291) -> ("Turb"=w290:u32)
            n144 = case shown="\"国弘\"" w310 {
              tunnel: [FALSE TRUE FALSE] -> w313
              tunnel: [0 ("y") 0 ("y") 36 ("y")] -> w305
              tunnel: [_ _ TRUE] -> w294
              tunnel: [_ w333 _] -> w293
              tunnel: [w326 w332 w347] -> w292
              tunnel: w290 -> [w326 _ w347]
              tunnel: [_ _ string[] ["（0-100）NTU", "（0-500）NTU", "（0-2000）NTU", "（0-4000）NTU"]] -> w289
              tunnel: [_ _ w344] -> w288
              tunnel: [_ w331 w342] -> w287
              tunnel: [_ TRUE TRUE] -> w286
              tunnel: [_ _ TRUE] -> w285
              tunnel: [_ _ TRUE] -> w284
              tunnel: [_ _ w339] -> w283
              tunnel: [_ _ w338] -> w282
              tunnel: [_ TRUE TRUE] -> w281
              frame "禹山", Default {
              }
              frame "国弘" {
                n145 = global read "国弘过程全局变量.vi" "Turb"() -> (w334:T11)
                n146 = Unbundle By Name(w334) -> ("命令滤波设定"=w332:u16, "浊度偏移修正值"=w333:sgl, "清洁周期"=w331:u16)
              }
              frame "纳清" {
                n147 = global read "纳清过程全局变量.vi" "浊度测试值"() -> (w345:T12)
                n148 = Unbundle By Name(w345) -> ("清扫模式"=w338:u16, "清扫次数"=w339:u16, "清扫间隔分钟"=w342:u16, "量程"=w344:u16)
              }
            }
            n149 = in-place {
              in-place-border: w305 -> [w317]
              n150 = in-place-cluster #18(T6 {"Left"=656, "Top"=185} ("位置 2")) -> ("Top"=w324:i32)
              n151 = in-place-cluster #19(T6 {"Left"=674, "Top"=256} ("位置 4")) -> ("Top"=w323:i32)
              n152 = in-place-cluster #20(T6 {"Left"=674, "Top"=221} ("位置 3")) -> ("Top"=w322:i32)
              n153 = in-place-cluster #21(T6 {"Left"=674, "Top"=149} ("位置")) -> ("Top"=w325:i32)
              n154 = in-place-cluster #22(T6 {"Left"=638, "Top"=366} ("位置 7")) -> ("Top"=w320:i32)
              n155 = in-place-cluster #23(T6 {"Left"=710, "Top"=328} ("位置 6")) -> ("Top"=w319:i32)
              n156 = in-place-cluster #24(T6 {"Left"=674, "Top"=292} ("位置 5")) -> ("Top"=w321:i32)
              n157 = Subtract(x=w322, y=w317) -> (x-y=w318:i32)
              n158 = in-place-cluster #18("Top"=w324) -> (w299:T6)
              n159 = in-place-cluster #19("Top"=w323) -> (w295:T6)
              n160 = in-place-cluster #20("Top"=w318) -> (w297:T6)
              n161 = in-place-cluster #21("Top"=w325) -> (w301:T6)
              n162 = in-place-cluster #22("Top"=w320) -> (w304:T6)
              n163 = in-place-cluster #23("Top"=w319) -> (w306:T6)
              n164 = in-place-cluster #24("Top"=w321) -> (w303:T6)
            }
          }
          frame 12 {
            n165 = Unbundle By Name(w352) -> ("悬浮物"=w351:u32)
            n166 = in-place {
              in-place-border: 0 ("y") -> [w374]
              n167 = in-place-cluster #25(T6 {"Left"=656, "Top"=185} ("位置 2")) -> ("Top"=w381:i32)
              n168 = in-place-cluster #26(T6 {"Left"=674, "Top"=256} ("位置 4")) -> ("Top"=w380:i32)
              n169 = in-place-cluster #27(T6 {"Left"=674, "Top"=221} ("位置 3")) -> ("Top"=w379:i32)
              n170 = in-place-cluster #28(T6 {"Left"=674, "Top"=149} ("位置")) -> ("Top"=w382:i32)
              n171 = in-place-cluster #29(T6 {"Left"=638, "Top"=366} ("位置 7")) -> ("Top"=w377:i32)
              n172 = in-place-cluster #30(T6 {"Left"=710, "Top"=328} ("位置 6")) -> ("Top"=w376:i32)
              n173 = in-place-cluster #31(T6 {"Left"=674, "Top"=292} ("位置 5")) -> ("Top"=w378:i32)
              n174 = Subtract(x=w379, y=w374) -> (x-y=w375:i32)
              n175 = in-place-cluster #25("Top"=w381) -> (w357:T6)
              n176 = in-place-cluster #26("Top"=w380) -> (w353:T6)
              n177 = in-place-cluster #27("Top"=w375) -> (w355:T6)
              n178 = in-place-cluster #28("Top"=w382) -> (w359:T6)
              n179 = in-place-cluster #29("Top"=w377) -> (w362:T6)
              n180 = in-place-cluster #30("Top"=w376) -> (w364:T6)
              n181 = in-place-cluster #31("Top"=w378) -> (w361:T6)
            }
          }
          frame 3 {
            n182 = Unbundle By Name(w386) -> ("Cond"=w385:u32)
            n183 = case shown="\"纳清\"" w404 {
              tunnel: [FALSE TRUE FALSE] -> w407
              tunnel: [0 ("y") 36 ("y") 72 ("y")] -> w399
              tunnel: [_ TRUE TRUE] -> w387
              tunnel: w385 -> [w419 _ w428]
              tunnel: [w419 w422 w428] -> w384
              tunnel: [_ w423 _] -> w383
              frame "禹山", Default {
              }
              frame "国弘" {
                n184 = global read "国弘过程全局变量.vi" "Cond"() -> (w424:T13)
                n185 = Unbundle By Name(w424) -> ("命令滤波设定"=w422:u16, "电导率偏移修正值"=w423:sgl)
              }
              frame "纳清" {
              }
            }
            n186 = in-place {
              in-place-border: w399 -> [w411]
              n187 = in-place-cluster #32(T6 {"Left"=656, "Top"=185} ("位置 2")) -> ("Top"=w417:i32)
              n188 = in-place-cluster #33(T6 {"Left"=674, "Top"=256} ("位置 4")) -> ("Top"=w416:i32)
              n189 = in-place-cluster #34(T6 {"Left"=674, "Top"=221} ("位置 3")) -> ("Top"=w410:i32)
              n190 = in-place-cluster #35(T6 {"Left"=674, "Top"=149} ("位置")) -> ("Top"=w418:i32)
              n191 = in-place-cluster #36(T6 {"Left"=638, "Top"=366} ("位置 7")) -> ("Top"=w414:i32)
              n192 = in-place-cluster #37(T6 {"Left"=710, "Top"=328} ("位置 6")) -> ("Top"=w413:i32)
              n193 = in-place-cluster #38(T6 {"Left"=674, "Top"=292} ("位置 5")) -> ("Top"=w415:i32)
              n194 = Subtract(x=w416, y=w411) -> (x-y=w412:i32)
              n195 = in-place-cluster #32("Top"=w417) -> (w393:T6)
              n196 = in-place-cluster #33("Top"=w412) -> (w389:T6)
              n197 = in-place-cluster #34("Top"=w410) -> (w391:T6)
              n198 = in-place-cluster #35("Top"=w418) -> (w395:T6)
              n199 = in-place-cluster #36("Top"=w414) -> (w398:T6)
              n200 = in-place-cluster #37("Top"=w413) -> (w400:T6)
              n201 = in-place-cluster #38("Top"=w415) -> (w397:T6)
            }
          }
          frame 4 {
            n202 = Unbundle By Name(w442) -> ("叶绿素a"=w441:u32)
            n203 = case shown="\"纳清\"" w459 {
              tunnel: [FALSE TRUE FALSE] -> w462
              tunnel: [0 ("y") 0 ("y") 36 ("y")] -> w454
              tunnel: [_ _ TRUE] -> w443
              tunnel: [_ _ string[] ["（0-500）μg/L", "（0-50）μg/L"]] -> w440
              tunnel: [_ _ w486] -> w439
              tunnel: [_ _ w485] -> w438
              tunnel: [_ _ w484] -> w437
              tunnel: [_ _ w483] -> w436
              tunnel: [_ _ TRUE] -> w435
              tunnel: [_ _ TRUE] -> w434
              tunnel: [_ _ TRUE] -> w433
              tunnel: [_ _ TRUE] -> w432
              frame "禹山", Default {
              }
              frame "国弘" {
              }
              frame "纳清" {
                n204 = global read "纳清过程全局变量.vi" "叶绿素a测试值"() -> (w487:T14)
                n205 = Unbundle By Name(w487) -> ("量程"=w486:u16, "清扫模式"=w485:u16, "清扫次数"=w484:u16, "清扫间隔分钟"=w483:u16)
              }
            }
            n206 = in-place {
              in-place-border: w454 -> [w466]
              n207 = in-place-cluster #39(T6 {"Left"=656, "Top"=185} ("位置 2")) -> ("Top"=w473:i32)
              n208 = in-place-cluster #40(T6 {"Left"=674, "Top"=256} ("位置 4")) -> ("Top"=w472:i32)
              n209 = in-place-cluster #41(T6 {"Left"=674, "Top"=221} ("位置 3")) -> ("Top"=w471:i32)
              n210 = in-place-cluster #42(T6 {"Left"=674, "Top"=149} ("位置")) -> ("Top"=w474:i32)
              n211 = in-place-cluster #43(T6 {"Left"=638, "Top"=366} ("位置 7")) -> ("Top"=w469:i32)
              n212 = in-place-cluster #44(T6 {"Left"=710, "Top"=328} ("位置 6")) -> ("Top"=w468:i32)
              n213 = in-place-cluster #45(T6 {"Left"=674, "Top"=292} ("位置 5")) -> ("Top"=w470:i32)
              n214 = Subtract(x=w471, y=w466) -> (x-y=w467:i32)
              n215 = in-place-cluster #39("Top"=w473) -> (w448:T6)
              n216 = in-place-cluster #40("Top"=w472) -> (w444:T6)
              n217 = in-place-cluster #41("Top"=w467) -> (w446:T6)
              n218 = in-place-cluster #42("Top"=w474) -> (w450:T6)
              n219 = in-place-cluster #43("Top"=w469) -> (w453:T6)
              n220 = in-place-cluster #44("Top"=w468) -> (w455:T6)
              n221 = in-place-cluster #45("Top"=w470) -> (w452:T6)
            }
          }
          frame 5 {
            n222 = Unbundle By Name(w502) -> ("藻密度"=w501:u32)
            n223 = case shown="\"纳清\"" w519 {
              tunnel: [FALSE TRUE FALSE] -> w522
              tunnel: [0 ("y") 0 ("y") 36 ("y")] -> w514
              tunnel: [_ _ TRUE] -> w503
              tunnel: [_ _ string[] ["（0-2000000）c/mL", "（0-200000）c/mL"]] -> w500
              tunnel: [_ _ w546] -> w499
              tunnel: [_ _ TRUE] -> w498
              tunnel: [_ _ w544] -> w497
              tunnel: [_ _ w543] -> w496
              tunnel: [_ _ w542] -> w495
              tunnel: [_ _ TRUE] -> w494
              tunnel: [_ _ TRUE] -> w493
              tunnel: [_ _ TRUE] -> w492
              frame "禹山", Default {
              }
              frame "国弘" {
              }
              frame "纳清" {
                n224 = global read "纳清过程全局变量.vi" "蓝绿藻测试值"() -> (w547:T15)
                n225 = Unbundle By Name(w547) -> ("量程"=w546:u16, "清扫模式"=w544:u16, "清扫次数"=w543:u16, "清扫间隔分钟"=w542:u16)
              }
            }
            n226 = in-place {
              in-place-border: w514 -> [w526]
              n227 = in-place-cluster #46(T6 {"Left"=656, "Top"=185} ("位置 2")) -> ("Top"=w533:i32)
              n228 = in-place-cluster #47(T6 {"Left"=674, "Top"=256} ("位置 4")) -> ("Top"=w532:i32)
              n229 = in-place-cluster #48(T6 {"Left"=674, "Top"=221} ("位置 3")) -> ("Top"=w531:i32)
              n230 = in-place-cluster #49(T6 {"Left"=674, "Top"=149} ("位置")) -> ("Top"=w534:i32)
              n231 = in-place-cluster #50(T6 {"Left"=638, "Top"=366} ("位置 7")) -> ("Top"=w529:i32)
              n232 = in-place-cluster #51(T6 {"Left"=710, "Top"=328} ("位置 6")) -> ("Top"=w528:i32)
              n233 = in-place-cluster #52(T6 {"Left"=674, "Top"=292} ("位置 5")) -> ("Top"=w530:i32)
              n234 = Subtract(x=w531, y=w526) -> (x-y=w527:i32)
              n235 = in-place-cluster #46("Top"=w533) -> (w508:T6)
              n236 = in-place-cluster #47("Top"=w532) -> (w504:T6)
              n237 = in-place-cluster #48("Top"=w527) -> (w506:T6)
              n238 = in-place-cluster #49("Top"=w534) -> (w510:T6)
              n239 = in-place-cluster #50("Top"=w529) -> (w513:T6)
              n240 = in-place-cluster #51("Top"=w528) -> (w515:T6)
              n241 = in-place-cluster #52("Top"=w530) -> (w512:T6)
            }
          }
          frame 6 {
            n242 = Unbundle By Name(w553) -> ("ORP"=w552:u32)
            n243 = case shown="\"国弘\"" w570 {
              tunnel: [FALSE TRUE] -> w573
              tunnel: [_ w588] -> w555
              tunnel: [w585 w587] -> w554
              tunnel: w552 -> [w585 _]
              frame "禹山", Default {
              }
              frame "国弘" {
                n244 = global read "国弘过程全局变量.vi" "ORP"() -> (w589:T16)
                n245 = Unbundle By Name(w589) -> ("命令滤波设定"=w587:u16, "偏移修正值"=w588:sgl)
              }
            }
            n246 = in-place {
              n247 = in-place-cluster #53(T6 {"Left"=656, "Top"=185} ("位置 2")) -> ("Top"=w583:i32)
              n248 = in-place-cluster #54(T6 {"Left"=674, "Top"=256} ("位置 4")) -> ("Top"=w582:i32)
              n249 = in-place-cluster #55(T6 {"Left"=674, "Top"=221} ("位置 3")) -> ("Top"=w581:i32)
              n250 = in-place-cluster #56(T6 {"Left"=674, "Top"=149} ("位置")) -> ("Top"=w584:i32)
              n251 = in-place-cluster #57(T6 {"Left"=638, "Top"=366} ("位置 7")) -> ("Top"=w578:i32)
              n252 = in-place-cluster #58(T6 {"Left"=710, "Top"=328} ("位置 6")) -> ("Top"=w579:i32)
              n253 = in-place-cluster #59(T6 {"Left"=674, "Top"=292} ("位置 5")) -> ("Top"=w580:i32)
              n254 = in-place-cluster #53("Top"=w583) -> (w560:T6)
              n255 = in-place-cluster #54("Top"=w582) -> (w556:T6)
              n256 = in-place-cluster #55("Top"=w581) -> (w558:T6)
              n257 = in-place-cluster #56("Top"=w584) -> (w562:T6)
              n258 = in-place-cluster #57("Top"=w578) -> (w565:T6)
              n259 = in-place-cluster #58("Top"=w579) -> (w566:T6)
              n260 = in-place-cluster #59("Top"=w580) -> (w564:T6)
            }
          }
          frame 7 {
            n261 = in-place {
              n262 = in-place-cluster #60(T6 {"Left"=656, "Top"=185} ("位置 2")) -> ("Top"=w620:i32)
              n263 = in-place-cluster #61(T6 {"Left"=674, "Top"=256} ("位置 4")) -> ("Top"=w619:i32)
              n264 = in-place-cluster #62(T6 {"Left"=674, "Top"=221} ("位置 3")) -> ("Top"=w618:i32)
              n265 = in-place-cluster #63(T6 {"Left"=674, "Top"=149} ("位置")) -> ("Top"=w621:i32)
              n266 = in-place-cluster #64(T6 {"Left"=638, "Top"=366} ("位置 7")) -> ("Top"=w615:i32)
              n267 = in-place-cluster #65(T6 {"Left"=710, "Top"=328} ("位置 6")) -> ("Top"=w616:i32)
              n268 = in-place-cluster #66(T6 {"Left"=674, "Top"=292} ("位置 5")) -> ("Top"=w617:i32)
              n269 = in-place-cluster #60("Top"=w620) -> (w598:T6)
              n270 = in-place-cluster #61("Top"=w619) -> (w594:T6)
              n271 = in-place-cluster #62("Top"=w618) -> (w596:T6)
              n272 = in-place-cluster #63("Top"=w621) -> (w600:T6)
              n273 = in-place-cluster #64("Top"=w615) -> (w603:T6)
              n274 = in-place-cluster #65("Top"=w616) -> (w604:T6)
              n275 = in-place-cluster #66("Top"=w617) -> (w602:T6)
            }
            n276 = global read "国弘过程全局变量.vi" "COD"() -> (w591:T17)
            n277 = Unbundle By Name(w591) -> ("数字滤波设定"=w593:u16, "COD偏移修正值"=w592:sgl)
          }
          frame 8 {
            n278 = Unbundle By Name(w626) -> ("DO"=w625:u32)
            n279 = case shown="\"禹山\", Default" w642 {
              tunnel: [FALSE TRUE] -> w645
              tunnel: [108 ("y") 72 ("y")] -> w637
              frame "禹山", Default {
              }
              frame "国弘" {
              }
            }
            n280 = in-place {
              in-place-border: w637 -> [w654]
              n281 = in-place-cluster #67(T6 {"Left"=656, "Top"=185} ("位置 2")) -> ("Top"=w652:i32)
              n282 = in-place-cluster #68(T6 {"Left"=674, "Top"=256} ("位置 4")) -> ("Top"=w651:i32)
              n283 = in-place-cluster #69(T6 {"Left"=674, "Top"=221} ("位置 3")) -> ("Top"=w650:i32)
              n284 = in-place-cluster #70(T6 {"Left"=674, "Top"=149} ("位置")) -> ("Top"=w653:i32)
              n285 = in-place-cluster #71(T6 {"Left"=638, "Top"=366} ("位置 7")) -> ("Top"=w658:i32)
              n286 = in-place-cluster #72(T6 {"Left"=710, "Top"=328} ("位置 6")) -> ("Top"=w660:i32)
              n287 = in-place-cluster #73(T6 {"Left"=674, "Top"=292} ("位置 5")) -> ("Top"=w656:i32)
              n288 = Subtract(x=w658, y=w654) -> (x-y=w657:i32)
              n289 = Subtract(x=w660, y=w654) -> (x-y=w659:i32)
              n290 = Subtract(x=w656, y=w654) -> (x-y=w655:i32)
              n291 = in-place-cluster #67("Top"=w652) -> (w631:T6)
              n292 = in-place-cluster #68("Top"=w651) -> (w627:T6)
              n293 = in-place-cluster #69("Top"=w650) -> (w629:T6)
              n294 = in-place-cluster #70("Top"=w653) -> (w633:T6)
              n295 = in-place-cluster #71("Top"=w657) -> (w636:T6)
              n296 = in-place-cluster #72("Top"=w659) -> (w638:T6)
              n297 = in-place-cluster #73("Top"=w655) -> (w635:T6)
            }
            n298 = global read "禹山过程全局变量.vi" "DO 2"() -> (w624:cluster{"温度测量值":sgl, "DO%":sgl, "DOmg/L":sgl})
            n299 = Unbundle By Name(w624) -> ("DOmg/L"=w623:sgl)
          }
          frame 9 {
            n300 = in-place {
              n301 = in-place-cluster #74(T6 {"Left"=656, "Top"=185} ("位置 2")) -> ("Top"=w694:i32)
              n302 = in-place-cluster #75(T6 {"Left"=674, "Top"=256} ("位置 4")) -> ("Top"=w693:i32)
              n303 = in-place-cluster #76(T6 {"Left"=674, "Top"=221} ("位置 3")) -> ("Top"=w692:i32)
              n304 = in-place-cluster #77(T6 {"Left"=674, "Top"=149} ("位置")) -> ("Top"=w695:i32)
              n305 = in-place-cluster #78(T6 {"Left"=638, "Top"=366} ("位置 7")) -> ("Top"=w689:i32)
              n306 = in-place-cluster #79(T6 {"Left"=710, "Top"=328} ("位置 6")) -> ("Top"=w690:i32)
              n307 = in-place-cluster #80(T6 {"Left"=674, "Top"=292} ("位置 5")) -> ("Top"=w691:i32)
              n308 = in-place-cluster #74("Top"=w694) -> (w672:T6)
              n309 = in-place-cluster #75("Top"=w693) -> (w668:T6)
              n310 = in-place-cluster #76("Top"=w692) -> (w670:T6)
              n311 = in-place-cluster #77("Top"=w695) -> (w674:T6)
              n312 = in-place-cluster #78("Top"=w689) -> (w677:T6)
              n313 = in-place-cluster #79("Top"=w690) -> (w678:T6)
              n314 = in-place-cluster #80("Top"=w691) -> (w676:T6)
            }
            n315 = global read "国弘过程全局变量.vi" "氯化物"() -> (w665:T18)
            n316 = Unbundle By Name(w665) -> ("命令滤波设定"=w667:u16, "偏移修正值"=w666:sgl)
          }
          frame 10 {
            n317 = Unbundle By Name(w696) -> ("氨氮"=w697:u32)
            n318 = in-place {
              n319 = in-place-cluster #81(T6 {"Left"=656, "Top"=185} ("位置 2")) -> ("Top"=w724:i32)
              n320 = in-place-cluster #82(T6 {"Left"=674, "Top"=256} ("位置 4")) -> ("Top"=w723:i32)
              n321 = in-place-cluster #83(T6 {"Left"=674, "Top"=221} ("位置 3")) -> ("Top"=w722:i32)
              n322 = in-place-cluster #84(T6 {"Left"=674, "Top"=149} ("位置")) -> ("Top"=w725:i32)
              n323 = in-place-cluster #85(T6 {"Left"=638, "Top"=366} ("位置 7")) -> ("Top"=w719:i32)
              n324 = in-place-cluster #86(T6 {"Left"=710, "Top"=328} ("位置 6")) -> ("Top"=w720:i32)
              n325 = in-place-cluster #87(T6 {"Left"=674, "Top"=292} ("位置 5")) -> ("Top"=w721:i32)
              n326 = in-place-cluster #81("Top"=w724) -> (w702:T6)
              n327 = in-place-cluster #82("Top"=w723) -> (w698:T6)
              n328 = in-place-cluster #83("Top"=w722) -> (w700:T6)
              n329 = in-place-cluster #84("Top"=w725) -> (w704:T6)
              n330 = in-place-cluster #85("Top"=w719) -> (w707:T6)
              n331 = in-place-cluster #86("Top"=w720) -> (w708:T6)
              n332 = in-place-cluster #87("Top"=w721) -> (w706:T6)
            }
          }
          frame 11 {
            n333 = in-place {
              in-place-border: 0 ("y") -> [w753]
              n334 = in-place-cluster #88(T6 {"Left"=656, "Top"=185} ("位置 2")) -> ("Top"=w760:i32)
              n335 = in-place-cluster #89(T6 {"Left"=674, "Top"=256} ("位置 4")) -> ("Top"=w759:i32)
              n336 = in-place-cluster #90(T6 {"Left"=674, "Top"=221} ("位置 3")) -> ("Top"=w758:i32)
              n337 = in-place-cluster #91(T6 {"Left"=674, "Top"=149} ("位置")) -> ("Top"=w761:i32)
              n338 = in-place-cluster #92(T6 {"Left"=638, "Top"=366} ("位置 7")) -> ("Top"=w756:i32)
              n339 = in-place-cluster #93(T6 {"Left"=710, "Top"=328} ("位置 6")) -> ("Top"=w755:i32)
              n340 = in-place-cluster #94(T6 {"Left"=674, "Top"=292} ("位置 5")) -> ("Top"=w757:i32)
              n341 = Subtract(x=w758, y=w753) -> (x-y=w754:i32)
              n342 = in-place-cluster #88("Top"=w760) -> (w736:T6)
              n343 = in-place-cluster #89("Top"=w759) -> (w732:T6)
              n344 = in-place-cluster #90("Top"=w754) -> (w734:T6)
              n345 = in-place-cluster #91("Top"=w761) -> (w738:T6)
              n346 = in-place-cluster #92("Top"=w756) -> (w741:T6)
              n347 = in-place-cluster #93("Top"=w755) -> (w743:T6)
              n348 = in-place-cluster #94("Top"=w757) -> (w740:T6)
            }
            n349 = global read "国弘过程全局变量.vi" "水中油"() -> (w726:T19)
            n350 = Unbundle By Name(w726) -> ("数位滤波设定"=w730:u16, "水中油B值"=w731:sgl, "清洁周期"=w729:u16)
          }
        }
        n351 = case shown="\"STD\"" w138 {
          tunnel: [TRUE TRUE FALSE TRUE] -> w137
          tunnel: [T5."Disabled and Grayed Out" ("禁用") T5."Enabled" ("禁用") T5."Enabled" ("禁用") T5."Enabled" ("禁用")] -> w136
          tunnel: [_ _ _ TRUE] -> w135
          frame "禹山", Default {
          }
          frame "国弘" {
          }
          frame "纳清" {
          }
          frame "STD" {
          }
        }
        n352 = property on="恢复出厂" class="Bool"("Visible"=w137) -> ()  [unwired: 2 in, 2 out]
        n353 = property on="KT" class="DigNum (strict)"("Visible"=w135) -> ()  [unwired: 2 in, 2 out]
        n354 = property on="BT" class="DigNum (strict)"("Visible"=w135) -> ()  [unwired: 2 in, 2 out]
        n355 = property on="校准温度" class="Bool"("DisabledEnum"=w136) -> ()  [unwired: 2 in, 2 out]
        n356 = property on="温度校准系数读取" class="Bool"("Visible"=w135) -> ()  [unwired: 2 in, 2 out]
        n357 = property on="温度校准系数写入" class="Bool"("Visible"=w135) -> ()  [unwired: 2 in, 2 out]
        n358 = global read "断电保存变量.vi" "大气压补偿"() -> (w154:dbl)
        n359 = global read "断电保存变量.vi" "盐度自动获取"() -> (w153:bool)
        n360 = property on="清洗选板" class="TabCtl (strict)"("Visible"=w141) -> ()  [unwired: 2 in, 2 out]
        n361 = property on="温度系数" class="DigNum (strict)"("Position"=w165, "Visible"=w158) -> ()  [unwired: 2 in, 2 out]
        n362 = property on="测量量程" class="Ring (strict)"("Position"=w166, "Visible"=w160, "Strings []"=w149, "Value"=w148) -> ()  [unwired: 2 in, 2 out]
        n363 = property on="滤波次数" class="DigNum (strict)"("Position"=w169, "Visible"=w161, "Value"=w152) -> ()  [unwired: 2 in, 2 out]
        n364 = property on="盐度" class="DigNum (strict)"("Position"=w163, "Visible"=w159) -> ()  [unwired: 2 in, 2 out]
        n365 = property on="清扫次数" class="DigNum (strict)"("Visible"=w145, "Value"=w143) -> ()  [unwired: 2 in, 2 out]
        n366 = property on="清扫间隔" class="DigNum (strict)"("Visible"=w146, "Value"=w147) -> ()  [unwired: 2 in, 2 out]
        n367 = property on="大气压力" class="DigNum (strict)"("Position"=w164, "Visible"=w155, "Value"=w154) -> ()  [unwired: 2 in, 2 out]
        n368 = property on="清扫模式" class="Ring (strict)"("Visible"=w144, "Value"=w142) -> ()  [unwired: 2 in, 2 out]
        n369 = property on="溶解氧浓度值" class="DigNum (strict)"("Visible"=w140, "Value"=w139) -> ()  [unwired: 2 in, 2 out]
        n370 = property on="偏移修正值" class="DigNum (strict)"("Position"=w167, "Visible"=w157, "Value"=w151) -> ()  [unwired: 2 in, 2 out]
        n371 = property on="自动盐度补偿" class="Bool (strict)"("Position"=w162, "Visible"=w156, "Value"=w153) -> ()  [unwired: 2 in, 2 out]
      }
    }
  }
  n372 = property on="窗格" class="Pane"("Origin"=T1 {"Horizontal"=0, "Vertical"=0} ("原点")) -> ()  [unwired: 2 in, 2 out]
  n373 = Create User Event(user event datatype=w5) -> (user event=w1:refnum<user-event>)  [unwired: 1 in, 1 out]
  n374 = global write "多参数全局变量.vi" "校准参数 event out"(w1) -> ()
  n375 = register-events(w1) -> (reference out=w4:refnum<event-registration>)  [unwired: 2 in, 1 out]
  n376 = Generate Occurrence() -> (w6:refnum<k4>)
  n377 = while {
    tunnel: w6 -> [w764]
    stop <- FALSE stop-if-true
    n378 = Wait on Occurrence(2:w764) -> (0:w762:bool)  [unwired: 2 in]
    n379 = flat-sequence {
      tunnel: w762 -> [_]
      frame #0 {
        n380 = call "信号曲线.vi"() -> ()  [unwired: 12 in]
      }
    }
  }
  n381 = while {
    tunnel: w6 -> [w767]
    tunnel: w4 -> [w766]
    tunnel: [w765] -> w3
    stop <- FALSE stop-if-true
    n382 = event shown="[1] <校准参数>: User Event" {
      selector: w766 -> [_ _ _ _ _ _ _ _ _ _ _ _ _ _ _ _ _ _ _ _ _ _]
      dyn-events: [_ _ _ _ _ _ _ _ _ _ _ _ _ _ _ _ _ _ _ _ _ _] -> w765
      timeout: _ -> [_ _ _ _ _ _ _ _ _ _ _ _ _ _ _ _ _ _ _ _ _ _]
      tunnel: w767 -> [_ _ _ _ w822 _ _ _ _ _ _ _ _ _ _ _ _ _ _ _ _ _]
      event Timeout {
        n383 = event-data() -> ()  [unwired: 1 in, 3 out]
      }
      event User Event {
        n384 = event-data() -> ("校准参数"=w769:u16)  [unwired: 1 in]
        n385 = property on="校准参数" class="Ring (strict)"("Val(Sgnl)"=w769) -> ()  [unwired: 2 in, 2 out]
      }
      event "温度校准系数读取": Value Change {
        # "悬浮物：已改"
        n386 = event-data() -> ()  [unwired: 1 in, 6 out]
        n387 = local read "校准参数"() -> (w779:u16)
        n388 = property on="校准参数" class="Ring (strict)"() -> ("Strings []"=w778:string[], "Value"=w777:u16)  [unwired: 2 in, 2 out]
        n389 = case shown="Default" w779 {
          tunnel: [T21."null" ("探头") T21."pH" ("探头") T21."DO" ("探头") T21."浊度" ("探头") T21."电导率" ("探头") T21."叶绿素a" ("探头") T21."DO2" ("探头") T21."藻密度" ("探头")] -> _
          frame Default {
          }
          frame 0 {
          }
          frame 1 {
          }
          frame 2 {
          }
          frame 3 {
          }
          frame 4 {
          }
          frame 5 {
          }
          frame 6 {
          }
        }
        n390 = Index Array(array=w778, index=w777) -> (element=w776:string)
        n391 = Search 1D Array(1D array=string[] ["null", "pH", "DO", "浊度", "电导率", "叶绿素a", "DO2", "藻密度", "悬浮物"] ("字符串[]"), element=w776) -> (index of element=w771:i32)  [unwired: 1 in]
        n392 = Equal?(x=w771, y=-1) -> (x = y?=w773:bool)
        n393 = global read "多参数全局变量.vi" "MB session in"() -> (w780:refnum<class "MB_Master.lvclass">)
        n394 = Select(t=T20."null" ("探头"), s=w773, f=w771) -> (s? t:f=w770:i32)
        n395 = call "STD获取温度校准参数.vi"("探头"=w770, "MB session in"=w780) -> ("error out"=w781:errorcluster, "输出值"=w785:cluster{"K":sgl, "B":sgl})  [unwired: 7 in, 1 out]
        n396 = case shown="No Error" w781 {
          tunnel: ["读取成功！" "读取失败！"] -> w782
          frame No Error {
          }
          frame Error {
          }
        }
        n397 = Unbundle By Name(w785) -> ("K"=w784:sgl, "B"=w783:sgl)
        n398 = local write "KT"(w784) -> ()
        n399 = local write "BT"(w783) -> ()
        n400 = One Button Dialog(message=w782) -> ()  [unwired: 1 in, 1 out]
      }
      event "温度校准系数写入": Value Change {
        # "悬浮物：已改"
        n401 = event-data() -> ()  [unwired: 1 in, 6 out]
        n402 = local read "校准参数"() -> (w807:u16)
        n403 = property on="校准参数" class="Ring (strict)"() -> ("Strings []"=w804:string[], "Value"=w803:u16)  [unwired: 2 in, 2 out]
        n404 = case shown="6" w807 {
          tunnel: [T21."null" ("探头") T21."pH" ("探头") T21."DO" ("探头") T21."浊度" ("探头") T21."电导率" ("探头") T21."叶绿素a" ("探头") T21."DO2" ("探头") T21."藻密度" ("探头")] -> _
          frame Default {
          }
          frame 0 {
          }
          frame 1 {
          }
          frame 2 {
          }
          frame 3 {
          }
          frame 4 {
          }
          frame 5 {
          }
          frame 6 {
          }
        }
        n405 = Index Array(array=w804, index=w803) -> (element=w802:string)
        n406 = Search 1D Array(1D array=string[] ["null", "pH", "DO", "浊度", "电导率", "叶绿素a", "DO2", "藻密度", "悬浮物"] ("字符串[]"), element=w802) -> (index of element=w797:i32)  [unwired: 1 in]
        n407 = Equal?(x=w797, y=-1) -> (x = y?=w799:bool)
        n408 = global read "多参数全局变量.vi" "MB session in"() -> (w808:refnum<class "MB_Master.lvclass">)
        n409 = Select(t=T20."null" ("探头"), s=w799, f=w797) -> (s? t:f=w796:i32)
        n410 = Bundle("KT"="KT", "BT"="BT") -> (w809:cluster{"KT":dbl, "BT":dbl})  [unwired: 1 in]
        n411 = call "STD设置温度校准参数.vi"("探头"=w796, "用户校准参数"=w809, "MB session in"=w808) -> ("error out"=w806:errorcluster)  [unwired: 7 in, 1 out]
        n412 = case shown="Error" w806 {
          tunnel: ["写入成功！" "写入失败！"] -> w805
          frame No Error {
          }
          frame Error {
          }
        }
        n413 = One Button Dialog(message=w805) -> ()  [unwired: 1 in, 1 out]
      }
      event "显示曲线": Value Change {
        n414 = event-data() -> ()  [unwired: 1 in, 6 out]
        n415 = Set Occurrence(w822) -> ()
      }
      event "温度系数": Value Change {
        n416 = event-data() -> ()  [unwired: 1 in, 6 out]
        n417 = property on="校准参数" class="Ring (strict)"() -> ("Value"=w826:u16)  [unwired: 2 in, 2 out]
        n418 = call "探头温度系数.vi"("校准参数"=w826, "温度系数"="温度系数") -> ("error out"=w823:errorcluster)  [unwired: 9 in]
        n419 = case shown="Error" w823 {
          tunnel: ["设置成功！" "设置失败！"] -> w824
          frame No Error {
          }
          frame Error {
          }
        }
        n420 = One Button Dialog(message=w824) -> ()  [unwired: 1 in, 1 out]
      }
      event "恢复出厂": Value Change {
        n421 = event-data() -> ()  [unwired: 1 in, 6 out]
        n422 = property on="校准参数" class="Ring (strict)"() -> ("Value"=w831:u16)  [unwired: 2 in, 2 out]
        n423 = call "探头恢复出厂.vi"("校准参数"=w831) -> ("error out"=w829:errorcluster)  [unwired: 10 in]
        n424 = case shown="Error" w829 {
          tunnel: ["设置成功！" "设置失败！"] -> w830
          frame No Error {
          }
          frame Error {
          }
        }
        n425 = One Button Dialog(message=w830) -> ()  [unwired: 1 in, 1 out]
      }
      event "测量量程": Value Change {
        n426 = event-data() -> ()  [unwired: 1 in, 6 out]
        n427 = property on="校准参数" class="Ring (strict)"() -> ("Value"=w836:u16)  [unwired: 2 in, 2 out]
        n428 = call "探头校准量程设置.vi"("校准参数"=w836, "校准量程"="测量量程") -> ("error out"=w835:errorcluster)  [unwired: 9 in]
        n429 = call "探头测量量程设置.vi"("校准参数"=w836, "error in (no error)"=w835, "测量量程设置"="测量量程") -> ("error out"=w837:errorcluster)  [unwired: 8 in]
        n430 = case shown="Error" w837 {
          tunnel: ["设置成功！" "设置失败！"] -> w838
          frame No Error {
          }
          frame Error {
          }
        }
        n431 = One Button Dialog(message=w838) -> ()  [unwired: 1 in, 1 out]
      }
      event "自动盐度补偿", "大气压力", "盐度", "滤波次数": Value Change {
        # "为什么？"
        n432 = event-data() -> ()  [unwired: 1 in, 6 out]
        n433 = flat-sequence {
          tunnel: [w842] -> w841
          tunnel: w841 -> [_]
          frame #0 {
            n434 = property on="校准参数" class="Ring (strict)"() -> ("Value"=w844:u16)  [unwired: 2 in, 2 out]
            n435 = global write "断电保存变量.vi" "盐度补偿"("盐度") -> ()
            n436 = global write "断电保存变量.vi" "大气压补偿"("大气压力") -> ()
            n437 = call "探头滤波次数.vi"("校准参数"=w844, "滤波次数"="滤波次数") -> ("error out"=w842:errorcluster)  [unwired: 9 in]
            n438 = global write "断电保存变量.vi" "盐度自动获取"("自动盐度补偿") -> ()
          }
          frame #1 {
            n439 = call "配置文件保存.vi"() -> ()  [unwired: 12 in]
          }
        }
      }
      event "清洗": Value Change {
        n440 = event-data() -> ()  [unwired: 1 in, 6 out]
        n441 = property on="校准参数" class="Ring (strict)"() -> ("Value"=w848:u16)  [unwired: 2 in, 2 out]
        n442 = call "探头手动清洗.vi"("校准参数"=w848) -> ("error out"=w849:errorcluster)  [unwired: 10 in]
        n443 = case shown="No Error" w849 {
          tunnel: ["启动成功！" "启动失败！"] -> w850
          frame No Error {
          }
          frame Error {
          }
        }
        n444 = One Button Dialog(message=w850) -> ()  [unwired: 1 in, 1 out]
      }
      event "清扫模式": Value Change {
        n445 = event-data() -> ()  [unwired: 1 in, 6 out]
        n446 = property on="校准参数" class="Ring (strict)"() -> ("Value"=w854:u16)  [unwired: 2 in, 2 out]
        n447 = case shown="12" w854 {
          tunnel: [T22."null" ("探头") T22."pH" ("探头") T22."DO" ("探头") T22."浊度" ("探头") T22."电导率" ("探头") T22."叶绿素a" ("探头") T22."藻密度" ("探头") 17 23] -> w853
          frame Default {
          }
          frame 0 {
          }
          frame 1 {
          }
          frame 2 {
          }
          frame 3 {
          }
          frame 4 {
          }
          frame 5 {
          }
          frame 11 {
          }
          frame 12 {
          }
        }
        n448 = call "纳清_清扫模式.vi"("探头"=w853, "清扫模式"="清扫模式") -> ("error out"=w855:errorcluster)  [unwired: 9 in]
        n449 = case shown="Error" w855 {
          tunnel: ["设置成功！" "设置失败！"] -> w856
          frame No Error {
          }
          frame Error {
          }
        }
        n450 = One Button Dialog(message=w856) -> ()  [unwired: 1 in, 1 out]
      }
      event "清扫次数": Value Change {
        n451 = event-data() -> ()  [unwired: 1 in, 6 out]
        n452 = property on="校准参数" class="Ring (strict)"() -> ("Value"=w873:u16)  [unwired: 2 in, 2 out]
        n453 = case shown="12" w873 {
          tunnel: [T22."null" ("探头") T22."pH" ("探头") T22."DO" ("探头") T22."浊度" ("探头") T22."电导率" ("探头") T22."叶绿素a" ("探头") T22."藻密度" ("探头") 17 23] -> w872
          frame Default {
          }
          frame 0 {
          }
          frame 1 {
          }
          frame 2 {
          }
          frame 3 {
          }
          frame 4 {
          }
          frame 5 {
          }
          frame 11 {
          }
          frame 12 {
          }
        }
        n454 = call "纳清_清扫次数.vi"("探头"=w872, "清扫次数"="清扫次数") -> ("error out"=w870:errorcluster)  [unwired: 9 in]
        n455 = case shown="Error" w870 {
          tunnel: ["设置成功！" "设置失败！"] -> w871
          frame No Error {
          }
          frame Error {
          }
        }
        n456 = One Button Dialog(message=w871) -> ()  [unwired: 1 in, 1 out]
      }
      event "清扫间隔": Value Change {
        n457 = event-data() -> ()  [unwired: 1 in, 6 out]
        n458 = property on="校准参数" class="Ring (strict)"() -> ("Value"=w886:u16)  [unwired: 2 in, 2 out]
        n459 = call "探头清洗间隔.vi"("校准参数"=w886, "清扫间隔"="清扫间隔") -> ("error out"=w885:errorcluster)  [unwired: 9 in]
        n460 = case shown="Error" w885 {
          tunnel: ["设置成功！" "设置失败！"] -> w888
          frame No Error {
          }
          frame Error {
          }
        }
        n461 = One Button Dialog(message=w888) -> ()  [unwired: 1 in, 1 out]
      }
      event "校准温度": Value Change {
        n462 = event-data() -> ()  [unwired: 1 in, 6 out]
        n463 = property on="校准参数" class="Ring (strict)"() -> ("Value"=w894:u16)  [unwired: 2 in, 2 out]
        n464 = call "温度校准.vi"("校准参数"=w894, "校准温度"="实际温度") -> ("error out"=w893:errorcluster)  [unwired: 9 in]
        n465 = case shown="Error" w893 {
          tunnel: ["校准成功！" "校准失败！"] -> w892
          frame No Error {
          }
          frame Error {
          }
        }
        n466 = One Button Dialog(message=w892) -> ()  [unwired: 1 in, 1 out]
      }
      event "偏移修正值": Value Change {
        n467 = event-data() -> ()  [unwired: 1 in, 6 out]
        n468 = property on="校准参数" class="Ring (strict)"() -> ("Value"=w898:u16)  [unwired: 2 in, 2 out]
        n469 = call "探头偏移修正值.vi"("校准参数"=w898, "温度偏移修正值"="偏移修正值") -> ("error out"=w899:errorcluster)  [unwired: 9 in]
        n470 = case shown="No Error" w899 {
          tunnel: ["设置成功！" "设置失败！"] -> w900
          frame No Error {
          }
          frame Error {
          }
        }
        n471 = One Button Dialog(message=w900) -> ()  [unwired: 1 in, 1 out]
      }
      event "标液一.标准值", "标液二.标准值", "标液三.标准值", "实际温度", "大气压力", "盐度", "滤波次数", "偏移修正值", "温度系数", "标液一.原始值", "标液三.原始值", "标液二.原始值": Mouse Down {
        n472 = event-data() -> ("CtlRef"=w906:refnum<vi>)  [unwired: 1 in, 7 out]
        n473 = property class="DigNum (strict)"(reference=w906) -> (reference out=w904:refnum<vi>, "Value"=w905:dbl)  [unwired: 1 in, 1 out]
        n474 = call "数字键盘.vi"("OldNumber"=w905) -> ("NewNumber"=w903:dbl)  [unwired: 1 in]
        n475 = property class="DigNum (strict)"(reference=w904, "Val(Sgnl)"=w903) -> ()  [unwired: 1 in, 2 out]
      }
      event "清扫次数", "清扫间隔": Mouse Down {
        n476 = event-data() -> ("CtlRef"=w910:refnum<vi>)  [unwired: 1 in, 7 out]
        n477 = property class="DigNum (strict)"(reference=w910) -> (reference out=w908:refnum<vi>, "Value"=w909:u16)  [unwired: 1 in, 1 out]
        n478 = call "数字键盘.vi"("OldNumber"=w909) -> ("NewNumber"=w907:dbl)  [unwired: 1 in]
        n479 = property class="DigNum (strict)"(reference=w908, "Val(Sgnl)"=w907) -> ()  [unwired: 1 in, 2 out]
      }
      event "标液一.标准值", "标液二.标准值", "标液三.标准值": Value Change {
        n480 = event-data() -> ()  [unwired: 1 in, 6 out]
        n481 = property on="校准参数" class="Ring (strict)"() -> ("Value"=w914:u16)  [unwired: 2 in, 2 out]
        n482 = property on="标准值" class="DigNum (strict)"() -> ("Value"=w913:dbl)  [unwired: 2 in, 2 out]
        n483 = property on="标准值" class="DigNum (strict)"() -> ("Value"=w912:dbl)  [unwired: 2 in, 2 out]
        n484 = property on="标准值" class="DigNum (strict)"() -> ("Value"=w911:dbl)  [unwired: 2 in, 2 out]
        n485 = call "探头校准标准值设置.vi"("校准参数"=w914, "标液三"=w911, "标液二"=w912, "标液一"=w913) -> ()  [unwired: 8 in]
      }
      event "校准参数": Value Change {
        n486 = event-data() -> ()  [unwired: 1 in, 6 out]
        n487 = property on="校准参数" class="Ring (strict)"() -> ("Value"=w917:u16)  [unwired: 2 in, 2 out]
        n488 = call "探头型号.vi"("校准参数"=w917) -> ("禁用项[]"=w916:i32[], "value"=w915:i32)  [unwired: 8 in, 1 out]
        n489 = property on="校准方式" class="Ring (strict)"("Disabled Items []"=w916, "Val(Sgnl)"=w915) -> ()  [unwired: 2 in, 2 out]
      }
      event "校准方式": Value Change {
        n490 = event-data() -> ()  [unwired: 1 in, 6 out]
        n491 = property on="校准参数" class="Ring (strict)"() -> ("Value"=w920:u16)  [unwired: 2 in, 2 out]
        n492 = call "探头型号.vi"("校准参数"=w920) -> ("探头型号"=w919:T3)  [unwired: 8 in, 2 out]
        n493 = case shown="\"禹山\", Default" w919 {
          tunnel: [_ TRUE] -> w918
          frame "禹山", Default {
          }
          frame "国弘" {
          }
        }
        n494 = flat-sequence {
          tunnel: w918 -> [w922]
          frame #0 {
            n495 = property on="校准方式" class="Ring (strict)"() -> ("Value"=w921:u16)  [unwired: 2 in, 2 out]
            n496 = case shown="2" w921 {
              tunnel: [cluster{bool, bool, bool} {TRUE, FALSE, FALSE} cluster{bool, bool, bool} {TRUE, TRUE, FALSE} cluster{bool, bool, bool} {TRUE, TRUE, TRUE}] -> w928
              frame 0, Default {
              }
              frame 1 {
              }
              frame 2 {
              }
            }
            n497 = Unbundle(w928) -> (w927:bool, w925:bool, w926:bool)
            n498 = property on="标液一" class="Clust (strict)"("Visible"=w927) -> ()  [unwired: 2 in, 2 out]
            n499 = property on="标液二" class="Clust (strict)"("Visible"=w925) -> ()  [unwired: 2 in, 2 out]
            n500 = property on="标液三" class="Clust (strict)"("Visible"=w926) -> ()  [unwired: 2 in, 2 out]
            n501 = And(x=w922, y=w925) -> (x .and. y?=w924:bool)
            n502 = And(x=w926, y=w922) -> (x .and. y?=w923:bool)
            n503 = property on="标液一开始校准" class="Bool (strict)"("Visible"=w927) -> ()  [unwired: 2 in, 2 out]
            n504 = property on="第一点确认校准" class="Bool"("Visible"=w927) -> ()  [unwired: 2 in, 2 out]
            n505 = property on="标液二开始校准" class="Bool (strict)"("Visible"=w925) -> ()  [unwired: 2 in, 2 out]
            n506 = property on="标液三开始校准" class="Bool (strict)"("Visible"=w926) -> ()  [unwired: 2 in, 2 out]
            n507 = property on="第二点确认校准" class="Bool"("Visible"=w924) -> ()  [unwired: 2 in, 2 out]
            n508 = property on="第三点确认校准" class="Bool"("Visible"=w923) -> ()  [unwired: 2 in, 2 out]
          }
        }
      }
      event "标液一开始校准", "标液二开始校准", "标液三开始校准": Value Change {
        n509 = event-data() -> ("CtlRef"=w945:refnum<vi>, "NewVal"=w934:bool)  [unwired: 1 in, 4 out]
        n510 = case shown="True" w934 {
          tunnel: [_ w947] -> w933
          frame False {
          }
          frame True {
            n511 = property on="校准参数" class="Ring (strict)"() -> ("Value"=w946:u16)  [unwired: 2 in, 2 out]
            n512 = case shown="8" w946 {
              tunnel: [T24 {"ph"=TRUE, "DO"=FALSE, "Cond"=FALSE, "Turb"=FALSE, "叶绿素a"=FALSE, "藻密度"=FALSE, "ORP"=FALSE, "COD"=FALSE, "DO2"=FALSE, FALSE, "氨氮"=FALSE, "水中油"=FALSE, "悬浮物"=FALSE, "余氯"=FALSE} ("校准运行状态") T24 {"ph"=FALSE, "DO"=TRUE, "Cond"=FALSE, "Turb"=FALSE, "叶绿素a"=FALSE, "藻密度"=FALSE, "ORP"=FALSE, "COD"=FALSE, "DO2"=FALSE, FALSE, "氨氮"=FALSE, "水中油"=FALSE, "悬浮物"=FALSE, "余氯"=FALSE} ("校准运行状态") T24 {"ph"=FALSE, "DO"=FALSE, "Cond"=FALSE, "Turb"=TRUE, "叶绿素a"=FALSE, "藻密度"=FALSE, "ORP"=FALSE, "COD"=FALSE, "DO2"=FALSE, FALSE, "氨氮"=FALSE, "水中油"=FALSE, "悬浮物"=FALSE, "余氯"=FALSE} ("校准运行状态") T24 {"ph"=FALSE, "DO"=FALSE, "Cond"=TRUE, "Turb"=FALSE, "叶绿素a"=FALSE, "藻密度"=FALSE, "ORP"=FALSE, "COD"=FALSE, "DO2"=FALSE, FALSE, "氨氮"=FALSE, "水中油"=FALSE, "悬浮物"=FALSE, "余氯"=FALSE} ("校准运行状态") T24 {"ph"=FALSE, "DO"=FALSE, "Cond"=FALSE, "Turb"=FALSE, "叶绿素a"=TRUE, "藻密度"=FALSE, "ORP"=FALSE, "COD"=FALSE, "DO2"=FALSE, FALSE, "氨氮"=FALSE, "水中油"=FALSE, "悬浮物"=FALSE, "余氯"=FALSE} ("校准运行状态") T24 {"ph"=FALSE, "DO"=FALSE, "Cond"=FALSE, "Turb"=FALSE, "叶绿素a"=FALSE, "藻密度"=TRUE, "ORP"=FALSE, "COD"=FALSE, "DO2"=FALSE, FALSE, "氨氮"=FALSE, "水中油"=FALSE, "悬浮物"=FALSE, "余氯"=FALSE} ("校准运行状态") T24 {"ph"=FALSE, "DO"=FALSE, "Cond"=FALSE, "Turb"=FALSE, "叶绿素a"=FALSE, "藻密度"=FALSE, "ORP"=TRUE, "COD"=FALSE, "DO2"=FALSE, FALSE, "氨氮"=FALSE, "水中油"=FALSE, "悬浮物"=FALSE, "余氯"=FALSE} ("校准运行状态") T24 {"ph"=FALSE, "DO"=FALSE, "Cond"=FALSE, "Turb"=FALSE, "叶绿素a"=FALSE, "藻密度"=FALSE, "ORP"=FALSE, "COD"=TRUE, "DO2"=FALSE, FALSE, "氨氮"=FALSE, "水中油"=FALSE, "悬浮物"=FALSE, "余氯"=FALSE} ("校准运行状态") T24 {"ph"=FALSE, "DO"=FALSE, "Cond"=FALSE, "Turb"=FALSE, "叶绿素a"=FALSE, "藻密度"=FALSE, "ORP"=FALSE, "COD"=FALSE, "DO2"=TRUE, FALSE, "氨氮"=FALSE, "水中油"=FALSE, "悬浮物"=FALSE, "余氯"=FALSE} ("校准运行状态") T24 {"ph"=FALSE, "DO"=FALSE, "Cond"=FALSE, "Turb"=FALSE, "叶绿素a"=FALSE, "藻密度"=FALSE, "ORP"=FALSE, "COD"=FALSE, "DO2"=FALSE, TRUE, "氨氮"=FALSE, "水中油"=FALSE, "悬浮物"=FALSE, "余氯"=FALSE} ("校准运行状态") T24 {"ph"=FALSE, "DO"=FALSE, "Cond"=FALSE, "Turb"=FALSE, "叶绿素a"=FALSE, "藻密度"=FALSE, "ORP"=FALSE, "COD"=FALSE, "DO2"=FALSE, FALSE, "氨氮"=TRUE, "水中油"=FALSE, "悬浮物"=FALSE, "余氯"=FALSE} ("校准运行状态") T24 {"ph"=FALSE, "DO"=FALSE, "Cond"=FALSE, "Turb"=FALSE, "叶绿素a"=FALSE, "藻密度"=FALSE, "ORP"=FALSE, "COD"=FALSE, "DO2"=FALSE, FALSE, "氨氮"=FALSE, "水中油"=TRUE, "悬浮物"=FALSE, "余氯"=FALSE} ("校准运行状态") T24 {"ph"=FALSE, "DO"=FALSE, "Cond"=FALSE, "Turb"=FALSE, "叶绿素a"=FALSE, "藻密度"=FALSE, "ORP"=FALSE, "COD"=FALSE, "DO2"=FALSE, FALSE, "氨氮"=FALSE, "水中油"=FALSE, "悬浮物"=TRUE, "余氯"=FALSE} ("校准运行状态")] -> w947
              frame 0, Default {
              }
              frame 1 {
              }
              frame 2 {
              }
              frame 3 {
              }
              frame 4 {
              }
              frame 5 {
              }
              frame 6 {
              }
              frame 7 {
              }
              frame 8 {
              }
              frame 9 {
              }
              frame 10 {
              }
              frame 11 {
              }
              frame 12 {
              }
            }
          }
        }
        n513 = property class="Bool (strict)"(reference=w945) -> ("Label.Text"=w944:string)  [unwired: 1 in, 2 out]
        n514 = case shown="\"标液三开始校准\"" w944 {
          tunnel: [w962 w964 w966] -> _
          tunnel: [T23 {"禁用"=enum."Enabled", "禁用 2"=enum."Disabled and Grayed Out", "禁用 3"=enum."Disabled and Grayed Out"} T23 {"禁用"=enum."Disabled and Grayed Out", "禁用 2"=enum."Enabled", "禁用 3"=enum."Disabled and Grayed Out"} T23 {"禁用"=enum."Disabled and Grayed Out", "禁用 2"=enum."Disabled and Grayed Out", "禁用 3"=enum."Enabled"}] -> w942
          frame "标液一开始校准", Default {
            w962 = u16 0 items=["第一点", "第二点", "第三点"] ("当前校准点位")
          }
          frame "标液二开始校准" {
            w964 = u16 1 items=["第一点", "第二点", "第三点"] ("当前校准点位")
          }
          frame "标液三开始校准" {
            w966 = u16 2 items=["第一点", "第二点", "第三点"] ("当前校准点位")
          }
        }
        n515 = Select(t=T5."Disabled and Grayed Out" ("禁用 3"), s=w934, f=T5."Enabled") -> (s? t:f=w935:T5)
        n516 = property on="校准参数" class="Ring (strict)"("DisabledEnum"=w935) -> ()  [unwired: 2 in, 2 out]
        n517 = property on="校准方式" class="Ring (strict)"("DisabledEnum"=w935) -> ()  [unwired: 2 in, 2 out]
        n518 = property on="第三点确认校准" class="Bool"("DisabledEnum"=w935) -> ()  [unwired: 2 in, 2 out]
        n519 = property on="第二点确认校准" class="Bool"("DisabledEnum"=w935) -> ()  [unwired: 2 in, 2 out]
        n520 = property on="第一点确认校准" class="Bool"("DisabledEnum"=w935) -> ()  [unwired: 2 in, 2 out]
        n521 = global write "多参数全局变量.vi" "校准运行状态"(w933) -> ()
        n522 = Select(t=w942, s=w934, f=T23 {"禁用"=enum."Enabled", "禁用 2"=enum."Enabled", "禁用 3"=enum."Enabled"}) -> (s? t:f=w941:T23)
        n523 = Unbundle(w941) -> ("禁用"=w943:T5, "禁用 2"=w937:T5, "禁用 3"=w936:T5)
        n524 = property on="标液一开始校准" class="Bool (strict)"("DisabledEnum"=w943) -> ()  [unwired: 2 in, 2 out]
        n525 = property on="标液二开始校准" class="Bool (strict)"("DisabledEnum"=w937) -> ()  [unwired: 2 in, 2 out]
        n526 = property on="标液三开始校准" class="Bool (strict)"("DisabledEnum"=w936) -> ()  [unwired: 2 in, 2 out]
      }
      event "第一点确认校准", "第二点确认校准", "第三点确认校准": Value Change {
        n527 = event-data() -> ("CtlRef"=w981:refnum<vi>)  [unwired: 1 in, 5 out]
        n528 = property on="校准参数" class="Ring (strict)"() -> ("Value"=w976:u16)  [unwired: 2 in, 2 out]
        n529 = call "探头型号.vi"("校准参数"=w976) -> ("探头型号"=w982:T3)  [unwired: 8 in, 2 out]
        n530 = property on="校准参数" class="Ring (strict)"() -> ("Value"=w974:u16)  [unwired: 2 in, 2 out]
        n531 = property on="校准方式" class="Ring (strict)"() -> ("Value"=w973:u16)  [unwired: 2 in, 2 out]
        n532 = case shown="\"禹山\", Default" w982 {
          tunnel: [w1009 w1021] -> w970
          tunnel: w981 -> [_ w1024]
          tunnel: [TRUE w1011] -> w975
          tunnel: w973 -> [_ w1022]
          tunnel: w974 -> [_ _]
          tunnel: [errorcluster {"status"=FALSE, "code"=0, "source"="校准成功！"} ("error in (no error)") w1013] -> w969
          tunnel: [errorcluster {"status"=TRUE, "code"=0, "source"="校准失败！"} ("error in (no error)") w1012] -> w968
          frame "禹山", Default {
            n533 = property on="校准方式" class="Ring (strict)"() -> ("Value"=w1009:u16)  [unwired: 2 in, 2 out]
          }
          frame "国弘" {
            n534 = property class="Bool"(reference=w1024) -> ("Label.Text"=w1023:string)  [unwired: 1 in, 2 out]
            n535 = case shown="\"第一点确认校准\", Default" w1023 {
              tunnel: [u16 0 ("Value") u16 1 ("Value") u16 2 ("Value")] -> w1021
              tunnel: ["第一点校准通过，请更换标液，准备第二点校准！" "第二点校准通过，请更换标液，准备第三点校准！" "校准成功！"] -> w1020
              tunnel: ["第一点校准失败，请重新校准！" "第二点校准失败，请重新校准！" "第三点校准失败，请重新校准！"] -> w1018
              frame "第一点确认校准", Default {
              }
              frame "第二点确认校准" {
              }
              frame "第三点确认校准" {
              }
            }
            n536 = Equal?(x=w1022, y=w1021) -> (x = y?=w1011:bool)
            n537 = Select(t="校准成功！", s=w1011, f=w1020) -> (s? t:f=w1016:string)
            n538 = Select(t="校准失败！", s=w1011, f=w1018) -> (s? t:f=w1015:string)
            n539 = Bundle By Name(cluster=errorcluster {"status"=FALSE, "code"=0, "source"="校准成功！"} ("error in (no error)"), "source"=w1016) -> (w1013:errorcluster)
            n540 = Bundle By Name(cluster=errorcluster {"status"=TRUE, "code"=0, "source"="校准失败！"} ("error in (no error)"), "source"=w1015) -> (w1012:errorcluster)
          }
        }
        n541 = property on="测量量程" class="Ring (strict)"() -> ("Value"=w967:u16)  [unwired: 2 in, 2 out]
        n542 = property on="标液一" class="Clust (strict)"() -> ("Value"=w979:cluster{"标准值":dbl, "检测值":dbl, "原始值":dbl})  [unwired: 2 in, 2 out]
        n543 = property on="标液二" class="Clust (strict)"() -> ("Value"=w978:cluster{"标准值":dbl, "检测值":dbl, "原始值":dbl})  [unwired: 2 in, 2 out]
        n544 = property on="标液三" class="Clust (strict)"() -> ("Value"=w977:cluster{"标准值":dbl, "检测值":dbl, "原始值":dbl})  [unwired: 2 in, 2 out]
        n545 = call "执行校准.vi"("校准点位"=w970, "校准方式"=w973, "校准量程"=w967, "校准参数"=w974, "标液三"=w977, "标液二"=w978, "标液一"=w979) -> ("error out"=w972:errorcluster)  [unwired: 4 in]
        n546 = case shown="No Error" w972 {
          selector: w972 -> [_ w1004]
          tunnel: [w997 "校准失败！"] -> w980
          tunnel: [w998 w1004] -> w971
          tunnel: w969 -> [w996 _]
          tunnel: w968 -> [w995 _]
          frame No Error {
            n547 = flat-sequence {
              tunnel: [w1001] -> w999
              frame #0 {
                n548 = Wait (ms)(milliseconds to wait=u32 2000 ("等待时间（毫秒）")) -> ()  [unwired: 1 out]
              }
              frame #1 {
                n549 = property on="电极状态标志" class="DigNum (strict)"() -> ("Value"=w1002:u16)  [unwired: 2 in, 2 out]
                n550 = case shown="0..2, 31..33" w1002 {
                  tunnel: [_ TRUE] -> w1001
                  frame Default {
                  }
                  frame 0..2, 31..33 {
                  }
                }
              }
            }
            n551 = Select(t=w996, s=w999, f=w995) -> (s? t:f=w998:errorcluster)
            n552 = Unbundle By Name(w998) -> ("source"=w997:string)
          }
          frame Error {
          }
        }
        n553 = One Button Dialog(message=w980) -> ()  [unwired: 1 in, 1 out]
        n554 = case shown="True" w975 {
          tunnel: w979 -> [_ w994]
          tunnel: w978 -> [_ w993]
          tunnel: w977 -> [_ w992]
          tunnel: w974 -> [_ w983]
          tunnel: w973 -> [_ w987]
          tunnel: w971 -> [_ w991]
          frame False {
          }
          frame True {
            n555 = call "探头测量值显示.vi"("校准参数"=w983) -> ("线性系数"=w986:cluster{bool, "K":sgl, "B":sgl})  [unwired: 3 in, 7 out]
            n556 = Unbundle By Name(w986) -> ("K"=w985:sgl, "B"=w984:sgl)
            n557 = control-ref of="校准记录"() -> (w989:refnum<vi>)
            n558 = property on="当前温度" class="DigNum (strict)"() -> ("Value"=w990:dbl)  [unwired: 2 in, 2 out]
            n559 = property on="序列号" class="Str"() -> ("Value"=w988:string)  [unwired: 2 in, 2 out]
            n560 = call "生成校准记录.vi"("标液一"=w994, "校准参数"=w983, "校准方式"=w987, "校准记录"=w989, "标液二"=w993, "标液三"=w992, "当前温度"=w990, "error in (no error)"=w991, "序列号"=w988, "K"=w985, "B"=w984) -> ()  [unwired: 3 in, 2 out]
          }
        }
      }
    }
  }
  n561 = Unregister For Events(event registration refnum=w3) -> (error out=w2:errorcluster)  [unwired: 1 in]
  n562 = Destroy User Event(user event=w1, error in=w2) -> ()  [unwired: 1 out]
